vi "AES Decrypt.vi"(0 "Password.In":string, 2 "BitKeyType(256)":u16(ring)=256 items=["AES bit key 128"=128, "AES bit key 192"=192, "AES bit key 256"=256], 7 "EncryptedText.In":string, 11 "error in":errorcluster, 13 "nonce":u32=123456789) -> (8 "DecryptedText.Out":string, 15 "error out":errorcluster)   [LabVIEW 2011]
doc: "AES.Decrypt VI takes string encrypted with Advanced Encryption Standart (AES) and decrypts it into initial text. \nAES.Decrypt.vi allows reentrant execution.\n-------------------------------------------------------------------------------------------\nThis VI belongs to Server Lab tools at Labicom.net (www.labicom.net) project of remote and virtual laboratories, written by (c) Igor Titov, 2011."
panel:
  in  "Product information, copyright notice, list of conditions and disclaimer":string="Please visit http://www.labicom.net to learn about remote and virtual laboratories. With it's services and tools you can create remote and/or virtual laboratory and even make money on it.\n \nCopyright (C) 2011 Igor Titov igor.ev.titov@gmail.com\n\nAll rights reserved.\n\nRedistribution and use without modification, are permitted provided that the following conditions are met:\n\n    * Redistributions of source code must retain the above copyright notice, this list of conditions and the following disclaimer.\n    * Redistributions of source code and in binary form may be freely used in all sorts of projects (including commercial ones). It is not obligatory to place copyright notice, this list of conditions and the following disclaimer in your product but you must mention the source (www.labicom.net, Igor Titov) on the web-site of the product.\n    * Neither the name of \"Labicom\", \"labicom.net\", \"Igor Titov\", nor the names of its contributors may be used to endorse or promote products derived from this software without specific prior written permission (except in situations mentioned in the terms and conditions of use of the \"Labicom\").\n\nTHIS SOFTWARE IS PROVIDED BY THE COPYRIGHT HOLDERS AND CONTRIBUTORS \"AS IS\" AND ANY EXPRESS OR IMPLIED WARRANTIES, INCLUDING, BUT NOT LIMITED TO, THE IMPLIED WARRANTIES OF MERCHANTABILITY AND FITNESS FOR A PARTICULAR PURPOSE ARE DISCLAIMED. IN NO EVENT SHALL THE COPYRIGHT OWNER OR CONTRIBUTORS BE LIABLE FOR ANY DIRECT, INDIRECT, INCIDENTAL, SPECIAL, EXEMPLARY, OR CONSEQUENTIAL DAMAGES (INCLUDING, BUT NOT LIMITED TO, PROCUREMENT OF SUBSTITUTE GOODS OR SERVICES; LOSS OF USE, DATA, OR PROFITS; OR BUSINESS INTERRUPTION) HOWEVER CAUSED AND ON ANY THEORY OF LIABILITY, \nWHETHER IN CONTRACT, STRICT LIABILITY, OR TORT (INCLUDING NEGLIGENCE OR OTHERWISE) ARISING IN ANY WAY OUT OF THE USE OF THIS SOFTWARE, EVEN IF ADVISED OF THE POSSIBILITY OF SUCH DAMAGE. "
  in  "Decipher Phases":enum16{"Logical Shifts", "Combine Bytes"}(ring)
  in  "Decrypt Phases":enum16{"Init", "Decipher"}(ring)
  out "unsigned byte.utf8":u8[](array[numeric])
  out "unsigned byte.text":u8[](array[numeric])
  out "plaintxtByte":i32[](array[numeric])
  out "ciphertextArr":string[](array[string])
  out "ct":string[](array[string])
  out "nBlocks":i32
  out "cipherCntr":u16[](array[numeric])
  in  "0x100000000":u64=4294967296 format="%.0x"
  in  "blockSize":i32=16
  out "keySchedule":u32[](array[numeric])
  out "ctrTxt":string
  out "counterBlock":u32[](array[numeric])
  out "nonceSec":u32
  out "nonceMs":u32
  out "pwBytes":u32[](array[numeric])
  out "nBytes":i32
  # "Virtual & Remote Laboratories\nwww.labicom.net"
  # "Real lab at YOUR home"
  # "Number of bits used in the key (256 by default).\nThe longer a key, the higher level of protection\nat expence of processor and RAM usage."
  # "Advanced Encryption Standart (AES)\nAES.Decrypt 1.0"
  # "Receives Password in String format (plain text)"
  # "Receives encrypted text needed to be decrypted"
  # "Decrypted (plain) text"
  # "o?e?Ae§Oo??)y?B,UoV\"\nQoyµAv"
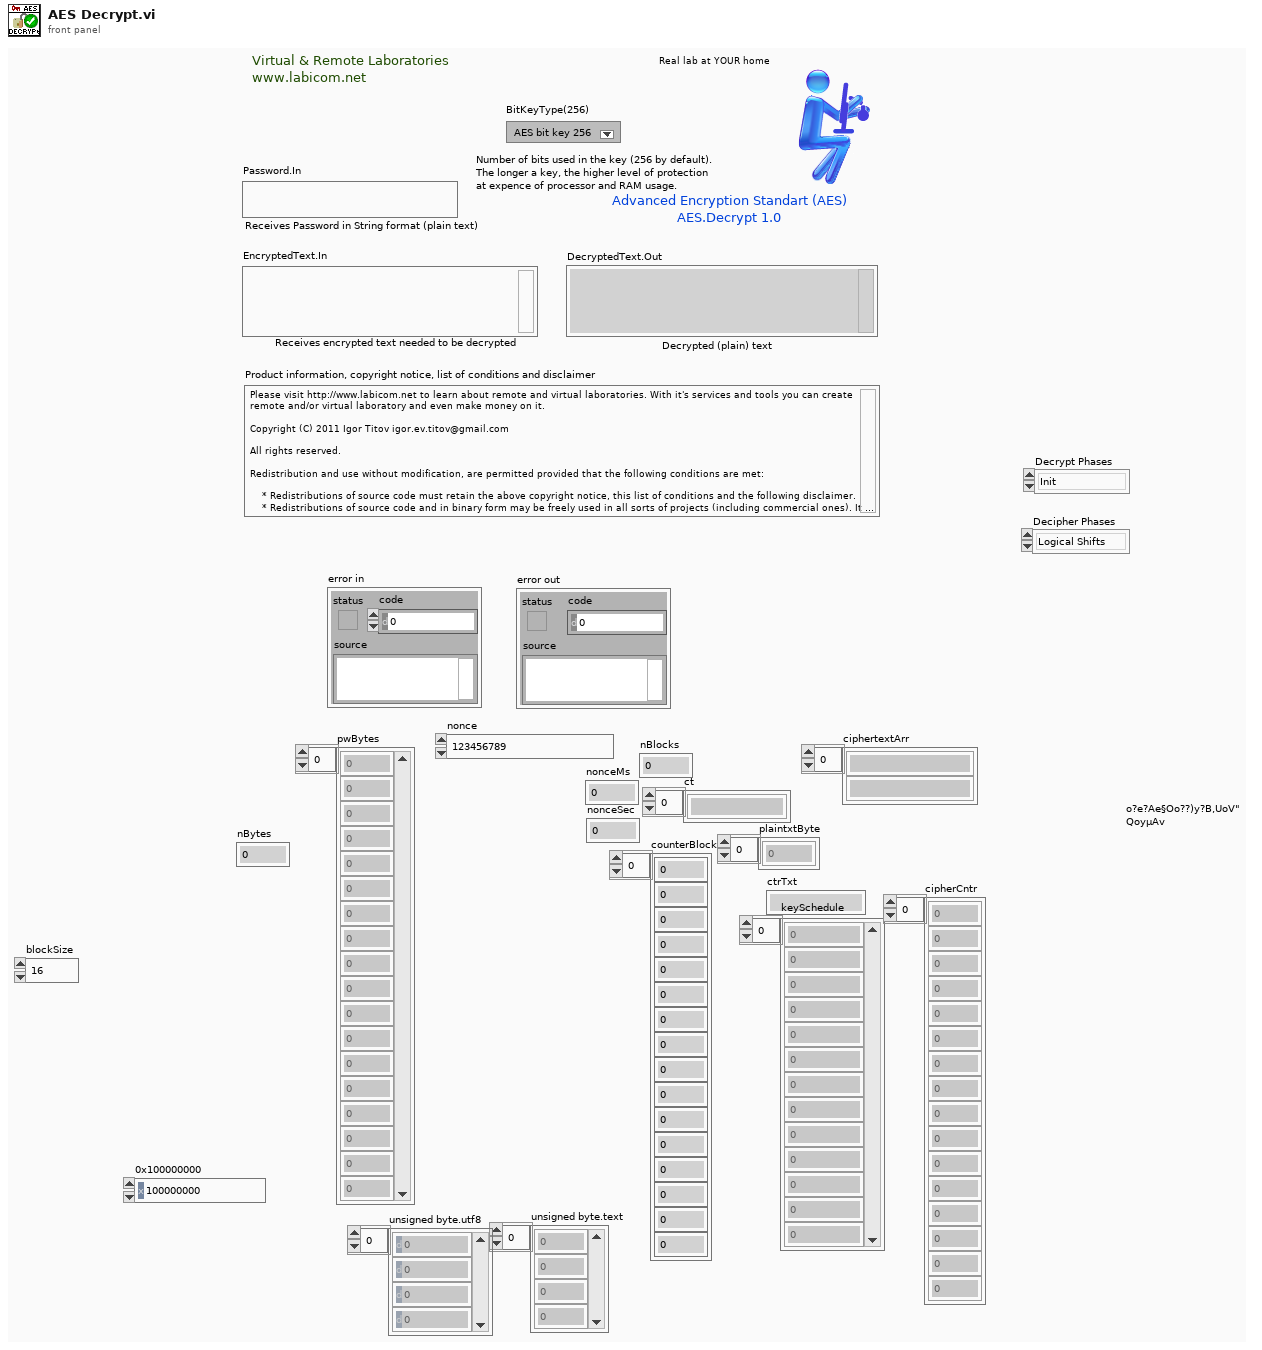
[diagram p1: front panel]
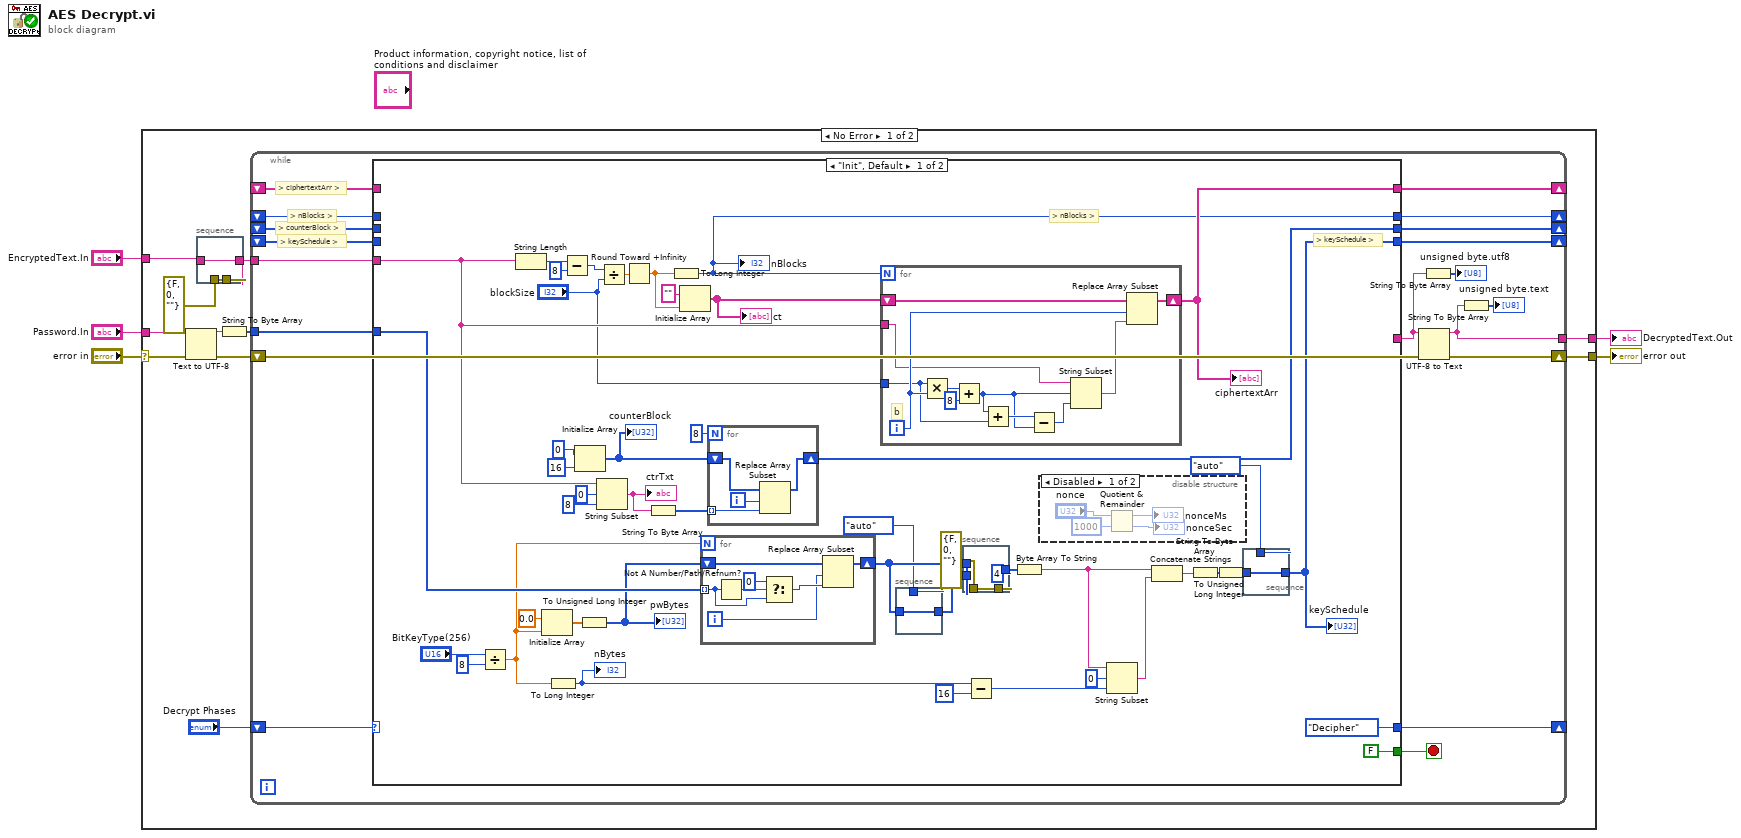
[diagram p0: block diagram]
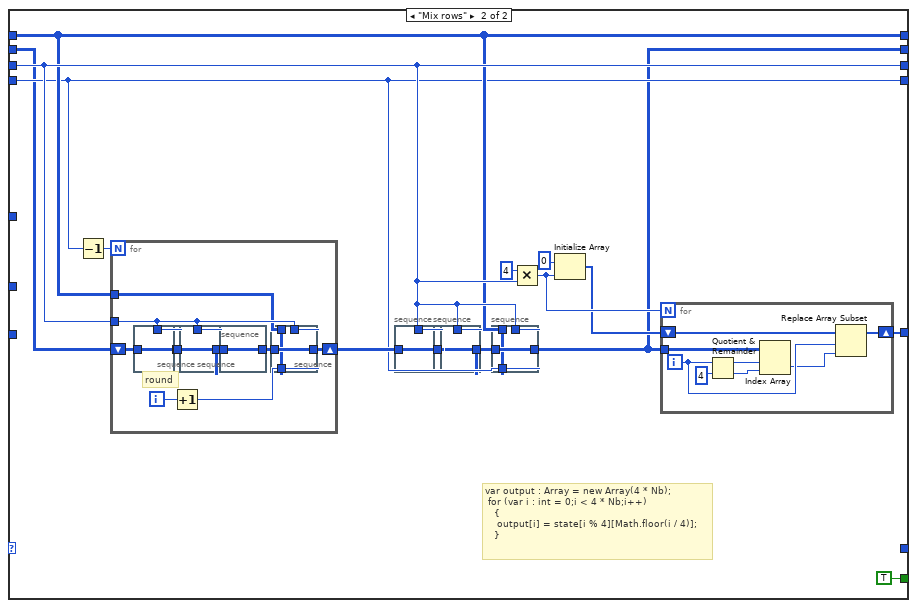
[diagram p2: hidden frame]
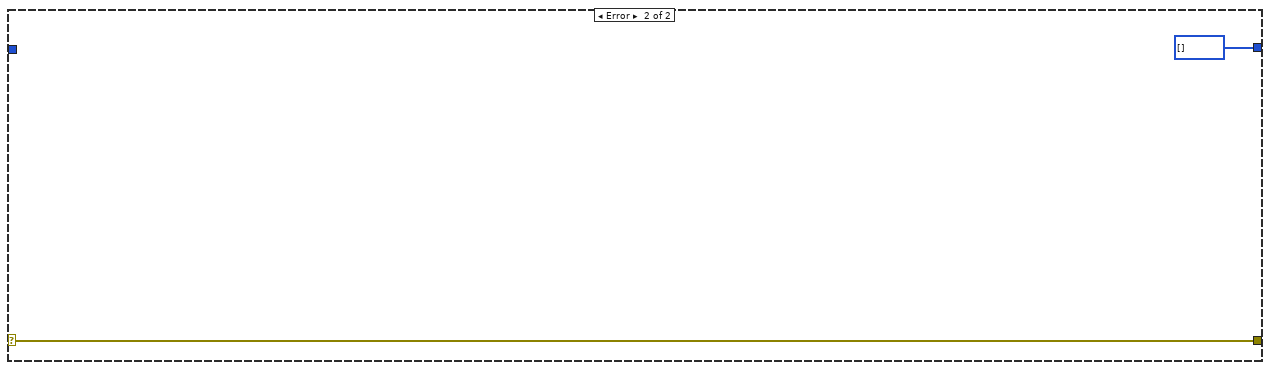
[diagram p3: hidden frame]
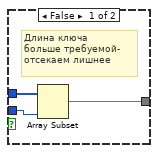
[diagram p4: hidden frame]
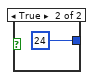
[diagram p5: hidden frame]
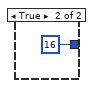
[diagram p6: hidden frame]
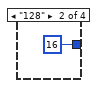
[diagram p7: hidden frame]
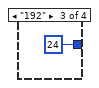
[diagram p8: hidden frame]
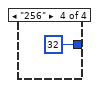
[diagram p9: hidden frame]
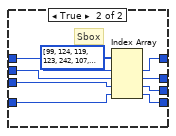
[diagram p10: hidden frame]
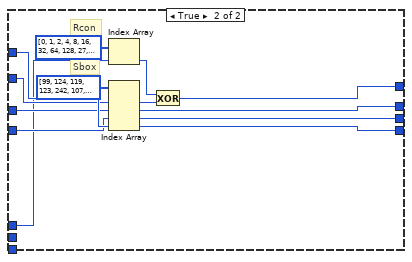
[diagram p11: hidden frame]
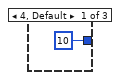
[diagram p12: hidden frame]
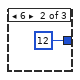
[diagram p13: hidden frame]
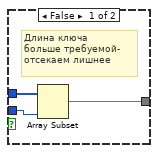
[diagram p14: hidden frame]
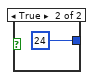
[diagram p15: hidden frame]
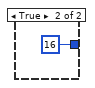
[diagram p16: hidden frame]
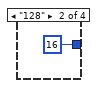
[diagram p17: hidden frame]
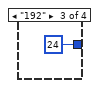
[diagram p18: hidden frame]
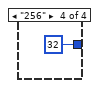
[diagram p19: hidden frame]
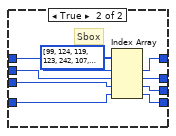
[diagram p20: hidden frame]
diagram:
  n1 = case shown="No Error" "error in" {
    selector: "error in" -> [w7 w1165]
    tunnel: [w12 w1165] -> w4
    tunnel: "EncryptedText.In" -> [w10 _]
    tunnel: "Password.In" -> [w9 _]
    tunnel: [w8 "" ("text")] -> w1
    frame No Error {
      n2 = Text to UTF-8(8:w7, 11:w9) -> (0:w11:errorcluster, 3:w15:string)
      n3 = stacked-sequence {
        tunnel: w10 -> [w28]
        tunnel: [w27] -> w13
        tunnel: errorcluster {"status"=FALSE, "code"=0, "source"=""} ("error in (no error)") -> [w35]
        tunnel: [w40] -> _
        frame #0 {
          w42 = TRUE ("replace all? (F)")
          w25 = 8 ("y")
          n4 = Search and Replace String(replace all?=w42, input string=w28, search string="\r" ("replace string (\"\")"), replace string="", error in=w35) -> (result string=w32:string, error out=w34:errorcluster)  [unwired: 5 out]
          n5 = Search and Replace String(replace all?=w42, input string=w32, search string="\n" ("replace string (\"\")"), replace string="", error in=w34) -> (result string=w38:string, error out=w39:errorcluster)  [unwired: 5 out]
          n6 = Search and Replace String(replace all?=w42, input string=w38, search string=" " ("replace string (\"\")"), replace string="", error in=w39) -> (result string=w41:string, error out=w40:errorcluster)  [unwired: 5 out]
          n7 = Match Pattern(string=w41, regular expression="=") -> (before substring=w20:string)  [unwired: 4 out]
          n8 = String Length(string=w20) -> (length=w17:i32)
          n9 = for {
            N: w17 -> [_]
            tunnel: w20 -> [w63]
            tunnel: "ABCDEFGHIJKLMNOPQRSTUVWXYZabcdefghijklmnopqrstuvwxyz0123456789+/" -> [w60]
            shift-right: [w53] -> w24
            shift-left: bool[] [] -> [w52]
            i -> [w61]
            n10 = String Subset(string=w63, offset (0)=w61, length (rest)=1 ("length (rest)")) -> (substring=w59:string)
            n11 = Match Pattern(string=w60, regular expression=w59) -> (offset past match=w58:i32)  [unwired: 1 in, 3 out]
            n12 = Decrement(x=w58) -> (x-1=w57:i32)
            n13 = Number To Boolean Array(number=w57) -> (Boolean array=w56:bool[])
            n14 = Array Subset(array=w56, length=6) -> (w54:bool[])  [unwired: 1 in]
            n15 = Reverse 1D Array(array=w54) -> (reversed array=w51:bool[])
            n16 = Build Array (concatenate)(w52, w51) -> (w53:bool[])
          }
          n17 = Array Size(array=w24) -> (size(s)=w22:i32)
          n18 = Quotient & Remainder(x=w22, y=w25) -> (floor(x/y)=w23:i32)  [unwired: 1 out]
          n19 = for {
            N: w23 -> [_]
            tunnel: w24 -> [w50]
            tunnel: w25 -> [w49]
            tunnel: [w45] -> w26 mode=indexing
            i -> [w48]
            n20 = Multiply(x=w48, y=w49) -> (x*y=w43:i32)
            n21 = Array Subset(array=w50, index=w43, length=w49) -> (w47:bool[])
            n22 = Reverse 1D Array(array=w47) -> (reversed array=w44:bool[])
            n23 = Boolean Array To Number(Boolean array=w44) -> (number=w46:u32)
            n24 = To Unsigned Byte Integer(number=w46) -> (unsigned 8bit integer=w45:u8)
          }
          n25 = Byte Array To String(unsigned byte array=w26) -> (string=w27:string)
        }
      }
      n26 = String To Byte Array(string=w15) -> (unsigned byte array=w14:u8[])
      n27 = while {
        shift-right: [w70] -> _
        shift-left: "Decrypt Phases" -> [w82]
        tunnel: w14 -> [w81]
        tunnel: w13 -> [w80]
        shift-right: [w78] -> _
        shift-left: _ -> [w77]
        shift-right: [w76] -> _
        shift-left: _ -> [w75]
        shift-right: [w74] -> _
        shift-left: _ -> [w73]
        shift-right: [w72] -> _
        shift-left: _ -> [w71]
        tunnel: [w66] -> w8
        shift-right: [w65] -> w12
        shift-left: w11 -> [w64]
        stop <- w79 stop-if-true
        # "> keySchedule >"
        # "> counterBlock >"
        # "> nBlocks >"
        # "> ciphertextArr >"
        n28 = case shown="\"Init\", Default" w82 {
          tunnel: w81 -> [w112 _]
          tunnel: w80 -> [w94 _]
          tunnel: [FALSE TRUE] -> w79
          tunnel: [w93 w758] -> w78
          tunnel: w77 -> [_ w758]
          tunnel: [w91 w759] -> w76
          tunnel: w75 -> [_ w759]
          tunnel: [w90 w760] -> w74
          tunnel: w73 -> [_ w760]
          tunnel: [w89 w762] -> w72
          tunnel: w71 -> [_ w762]
          tunnel: [enum16{"Init", "Decipher"}."Decipher" ("Decrypt Phases") _] -> w70
          tunnel: [_ w757] -> w67
          frame "Init", Default {
            # "> keySchedule >"
            # "> nBlocks >"
            n29 = Divide(x="BitKeyType(256)", y=u16 8) -> (x/y=w99:dbl)
            n30 = String Length(string=w94) -> (length=w121:i32)
            n31 = Initialize Array(0.0 ("element"), w99) -> (w111:dbl[])
            n32 = To Long Integer(number=w99) -> (32bit integer=w98:i32)
            "nBytes" <- w98
            n33 = Subtract(x=w121, y=8) -> (x-y=w119:i32)
            n34 = Initialize Array(u32 0 ("y"), 16 ("dimension size")) -> (w109:u32[])
            "counterBlock" <- w109
            n35 = To Unsigned Long Integer(number=w111) -> (unsigned 32bit integer=w110:u32[])
            "pwBytes" <- w110
            n36 = String Subset(string=w94, offset (0)=0, length (rest)=8 ("length (rest)")) -> (substring=w115:string)
            "ctrTxt" <- w115
            n37 = Divide(x=w119, y="blockSize") -> (x/y=w118:dbl)
            n38 = Round Toward +Infinity(x=w118) -> (ceil(x): smallest int >= x=w97:dbl)
            n39 = String To Byte Array(string=w115) -> (unsigned byte array=w116:u8[])
            n40 = To Long Integer(number=w97) -> (32bit integer=w91:i32)
            "nBlocks" <- w91
            n41 = Initialize Array("", w97) -> (w96:string[])
            "ct" <- w96
            n42 = for {
              N: w99 -> [_]
              tunnel: w112 -> [w751] mode=indexing
              shift-right: [w749] -> w100
              shift-left: w110 -> [w750]
              i -> [w753]
              n43 = Not A Number/Path/Refnum?(number/path/refnum=w751) -> (NaN/Path/Refnum?=w755:bool)
              n44 = Select(t=0 ("f"), s=w755, f=w751) -> (s? t:f=w754:i32)
              n45 = Replace Array Subset(array=w750, new element=w754, index=w753) -> (w749:u32[])
            }
            n46 = for {
              N: 8 -> [_]
              tunnel: w116 -> [w748] mode=indexing
              shift-right: [w745] -> w90
              shift-left: w109 -> [w746]
              i -> [w747]
              n47 = Replace Array Subset(array=w746, new element=w748, index=w747) -> (w745:u32[])
            }
            n48 = for {
              N: w91 -> [_]
              shift-right: [w736] -> w93
              shift-left: w96 -> [w737]
              tunnel: w94 -> [w735]
              tunnel: "blockSize" -> [w734]
              i -> [w742]
              # "b"
              n49 = Multiply(x=w734, y=w742) -> (x*y=w744:i32)
              n50 = Add(x=w744, y=8) -> (x+y=w739:i32)
              n51 = Add(x=w739, y=w734) -> (x+y=w740:i32)
              n52 = Subtract(x=w740, y=w739) -> (x-y=w738:i32)
              n53 = String Subset(string=w735, offset (0)=w739, length (rest)=w738) -> (substring=w741:string)
              n54 = Replace Array Subset(array=w737, new element=w741, index=w742) -> (w736:string[])
            }
            "ciphertextArr" <- w93
            n55 = stacked-sequence {
              tunnel: enum16{"128", "192", "256", "auto"}."auto" ("Mode (auto)") -> [w464]
              tunnel: w100 -> [w469]
              tunnel: [w470] -> w101
              frame #0 {
                n56 = Array Size(array=w469) -> (size(s)=w465:i32)
                n57 = case shown="\"auto\", Default" w464 {
                  tunnel: w465 -> [w479 _ _ _]
                  tunnel: [w480 16 24 32] -> w467
                  frame "auto", Default {
                    n58 = Less Or Equal?(x=w479, y=16) -> (x <= y?=w481:bool)
                    n59 = case shown="False" w481 {
                      tunnel: [w483 16] -> w480
                      tunnel: w479 -> [w486 _]
                      frame False {
                        n60 = Less Or Equal?(x=w486, y=24) -> (x <= y?=w484:bool)
                        n61 = case shown="False" w484 {
                          tunnel: [32 ("y") 24 ("y")] -> w483
                          frame False {
                          }
                          frame True {
                          }
                        }
                      }
                      frame True {
                      }
                    }
                  }
                  frame "128" {
                  }
                  frame "192" {
                  }
                  frame "256" {
                  }
                }
                n62 = Less?(x=w465, y=w467) -> (x < y?=w466:bool)
                n63 = case shown="True" w466 {
                  tunnel: w469 -> [w473 w474]
                  tunnel: w467 -> [w472 w478]
                  tunnel: [w471 w476] -> w468
                  frame False {
                    # "Длина ключа\nбольше требуемой-\nотсекаем лишнее"
                    n64 = Array Subset(array=w473, length=w472) -> (w471:u32[])  [unwired: 1 in]
                  }
                  frame True {
                    # "Длина ключа\nменьше требуемой-\nдополняем нулями"
                    n65 = Initialize Array(u32 0, w478) -> (w477:u32[])
                    n66 = Replace Array Subset(array=w477, new element=w474) -> (w476:u32[])  [unwired: 1 in]
                  }
                }
                n67 = Array Size(array=w468) -> (size(s)=w463:i32)
                n68 = Logical Shift(y=i8 -2, x=w463) -> (x << y=w456:i32)
                n69 = case shown="8" w456 {
                  tunnel: [10 12 14] -> w453
                  frame 4, Default {
                  }
                  frame 6 {
                  }
                  frame 8 {
                  }
                }
                n70 = Increment(x=w453) -> (x+1=w454:i32)
                n71 = Multiply(x=4, y=w454) -> (x*y=w460:i32)
                n72 = Logical Shift(y=i8 2, x=w460) -> (x << y=w459:i32)
                n73 = Initialize Array(u32 0 ("element"), w459) -> (w461:u32[])
                n74 = Replace Array Subset(array=w461, new element=w468) -> (w462:u32[])  [unwired: 1 in]
                n75 = while {
                  tunnel: w460 -> [w545]
                  tunnel: w456 -> [w525]
                  shift-right: [w502] -> w470
                  shift-left: w462 -> [w526]
                  tunnel: w467 -> [w524]
                  i -> [w546]
                  stop <- w544 continue-if-true
                  n76 = Add(x=w525, y=w546) -> (x+y=w528:i32)
                  n77 = Less?(x=w528, y=w545) -> (x < y?=w544:bool)
                  n78 = Quotient & Remainder(x=w528, y=w525) -> (x-y*floor(x/y)=w533:i32, floor(x/y)=w527:i32)
                  n79 = Logical Shift(y=i8 2, x=w528) -> (x << y=w497:i32)
                  n80 = Equal To 0?(x=w533) -> (x = 0?=w534:bool)
                  n81 = Subtract(x=w497, y=4) -> (x-y=w538:i32)
                  n82 = Subtract(x=w497, y=3) -> (x-y=w537:i32)
                  n83 = Subtract(x=w497, y=2) -> (x-y=w536:i32)
                  n84 = Subtract(x=w497, y=1) -> (x-y=w535:i32)
                  n85 = Index Array(array=w526, index #1=w538, index #2=w537, index #3=w536, index #4=w535) -> (element #1=w532:u32, element #2=w531:u32, element #3=w530:u32, element #4=w529:u32)
                  n86 = case shown="False" w534 {
                    tunnel: w525 -> [w561 _]
                    tunnel: w533 -> [w559 _]
                    tunnel: w532 -> [w554 w587]
                    tunnel: w531 -> [w553 w586]
                    tunnel: w530 -> [w552 w585]
                    tunnel: w529 -> [w551 w584]
                    tunnel: w527 -> [_ w583]
                    tunnel: [w550 w580] -> w506
                    tunnel: [w549 w579] -> w505
                    tunnel: [w548 w578] -> w504
                    tunnel: [w547 w577] -> w503
                    frame False {
                      n87 = Greater?(x=w561, y=6) -> (0:w557:bool)
                      n88 = Equal?(x=w559, y=4) -> (x = y?=w556:bool)
                      n89 = And(x=w557, y=w556) -> (x .and. y?=w555:bool)
                      n90 = case shown="False" w555 {
                        tunnel: w554 -> [w565 w574]
                        tunnel: w553 -> [w564 w573]
                        tunnel: w552 -> [w563 w572]
                        tunnel: w551 -> [w562 w571]
                        tunnel: [w565 w570] -> w550
                        tunnel: [w564 w569] -> w549
                        tunnel: [w563 w568] -> w548
                        tunnel: [w562 w567] -> w547
                        frame False {
                        }
                        frame True {
                          # "Sbox"
                          n91 = Index Array(array=u32[] [99, 124, 119, 123, 242, 107, 111, 197, 48, 1, 103, 43, 254, 215, 171, 118, 202, 130, 201, 125, 250, 89, 71, 240, 173, 212, 162, 175, 156, 164, 114, 192, 183, 253, 147, 38, 54, 63, 247, 204, 52, 165, 229, 241, 113, 216, 49, 21, 4, 199, 35, 195, 24, 150, 5, 154, 7, 18, 128, 226, 235, 39, 178, 117, 9, 131, 44, 26, 27, 110, 90, 160, 82, 59, 214, 179, 41, 227, 47, 132, 83, 209, 0, 237, 32, 252, 177, 91, 106, 203, 190, 57, 74, 76, 88, 207, 208, 239, 170, 251, 67, 77, 51, 133, 69, 249, 2, 127, 80, 60, 159, 168, 81, 163, 64, 143, 146, 157, 56, 245, 188, 182, 218, 33, 16, 255, 243, 210, 205, 12, 19, 236, 95, 151, 68, 23, 196, 167, 126, 61, 100, 93, 25, 115, 96, 129, 79, 220, 34, 42, 144, 136, 70, 238, 184, 20, 222, 94, 11, 219, 224, 50, 58, 10, 73, 6, 36, 92, 194, 211, 172, 98, 145, 149, 228, 121, 231, 200, 55, 109, 141, 213, 78, 169, 108, 86, 244, 234, 101, 122, 174, 8, 186, 120, 37, 46, 28, 166, 180, 198, 232, 221, 116, 31, 75, 189, 139, 138, 112, 62, 181, 102, 72, 3, 246, 14, 97, 53, 87, 185, 134, 193, 29, 158, 225, 248, 152, 17, 105, 217, 142, 148, 155, 30, 135, 233, 206, 85, 40, 223, 140, 161, 137, 13, 191, 230, 66, 104, 65, 153, 45, 15, 176, 84, 187, 22] ("Sbox"), index #1=w574, index #2=w573, index #3=w572, index #4=w571) -> (element #1=w570:u32, element #2=w569:u32, element #3=w568:u32, element #4=w567:u32)
                        }
                      }
                    }
                    frame True {
                      # "Sbox"
                      # "Rcon"
                      n92 = Index Array(array=u32[] [0, 1, 2, 4, 8, 16, 32, 64, 128, 27, 54] ("Rcon"), index=w583) -> (element=w582:u32)
                      n93 = Index Array(array=u32[] [99, 124, 119, 123, 242, 107, 111, 197, 48, 1, 103, 43, 254, 215, 171, 118, 202, 130, 201, 125, 250, 89, 71, 240, 173, 212, 162, 175, 156, 164, 114, 192, 183, 253, 147, 38, 54, 63, 247, 204, 52, 165, 229, 241, 113, 216, 49, 21, 4, 199, 35, 195, 24, 150, 5, 154, 7, 18, 128, 226, 235, 39, 178, 117, 9, 131, 44, 26, 27, 110, 90, 160, 82, 59, 214, 179, 41, 227, 47, 132, 83, 209, 0, 237, 32, 252, 177, 91, 106, 203, 190, 57, 74, 76, 88, 207, 208, 239, 170, 251, 67, 77, 51, 133, 69, 249, 2, 127, 80, 60, 159, 168, 81, 163, 64, 143, 146, 157, 56, 245, 188, 182, 218, 33, 16, 255, 243, 210, 205, 12, 19, 236, 95, 151, 68, 23, 196, 167, 126, 61, 100, 93, 25, 115, 96, 129, 79, 220, 34, 42, 144, 136, 70, 238, 184, 20, 222, 94, 11, 219, 224, 50, 58, 10, 73, 6, 36, 92, 194, 211, 172, 98, 145, 149, 228, 121, 231, 200, 55, 109, 141, 213, 78, 169, 108, 86, 244, 234, 101, 122, 174, 8, 186, 120, 37, 46, 28, 166, 180, 198, 232, 221, 116, 31, 75, 189, 139, 138, 112, 62, 181, 102, 72, 3, 246, 14, 97, 53, 87, 185, 134, 193, 29, 158, 225, 248, 152, 17, 105, 217, 142, 148, 155, 30, 135, 233, 206, 85, 40, 223, 140, 161, 137, 13, 191, 230, 66, 104, 65, 153, 45, 15, 176, 84, 187, 22] ("Sbox"), index #1=w586, index #2=w585, index #3=w584, index #4=w587) -> (element #1=w581:u32, element #2=w579:u32, element #3=w578:u32, element #4=w577:u32)
                      n94 = Exclusive Or(1:w581, 2:w582) -> (0:w580:u32)
                    }
                  }
                  n95 = Subtract(x=w497, y=w524) -> (x-y=w523:i32)
                  n96 = Add(x=w523, y=0) -> (x+y=w518:i32)
                  n97 = Add(x=w523, y=1) -> (x+y=w517:i32)
                  n98 = Add(x=w523, y=2) -> (x+y=w516:i32)
                  n99 = Add(x=w523, y=3) -> (x+y=w515:i32)
                  n100 = Index Array(array=w526, index #1=w518, index #2=w517, index #3=w516, index #4=w515) -> (element #1=w514:u32, element #2=w513:u32, element #3=w512:u32, element #4=w511:u32)
                  n101 = Exclusive Or(1:w506, 2:w514) -> (0:w510:u32)
                  n102 = Exclusive Or(1:w505, 2:w513) -> (0:w509:u32)
                  n103 = Exclusive Or(1:w504, 2:w512) -> (0:w508:u32)
                  n104 = Exclusive Or(1:w503, 2:w511) -> (0:w507:u32)
                  n105 = Add(x=w497, y=0) -> (x+y=w496:i32)
                  n106 = Add(x=w497, y=1) -> (x+y=w495:i32)
                  n107 = Add(x=w497, y=2) -> (x+y=w494:i32)
                  n108 = Add(x=w497, y=3) -> (x+y=w493:i32)
                  n109 = Replace Array Subset(array=w526, new element #1=w510, index #1=w496, new element #2=w509, index #2=w495, new element #3=w508, index #3=w494, new element #4=w507, index #4=w493) -> (w502:u32[])
                }
              }
            }
            n110 = stacked-sequence {
              tunnel: w100 -> [w131]
              tunnel: [w132] -> w102
              tunnel: w101 -> [w130]
              tunnel: errorcluster {"status"=FALSE, "code"=0, "source"=""} ("error in") -> [w128]
              tunnel: [w129] -> _
              frame #0 {
                n111 = case shown="No Error" w128 {
                  selector: w128 -> [_ w451]
                  tunnel: [_ w451] -> w129
                  tunnel: w130 -> [w137 _]
                  tunnel: w131 -> [w136 _]
                  tunnel: [w135 u16[] []] -> w132
                  tunnel: 4 ("Nb") -> [w134 _]
                  frame No Error {
                    n112 = while {
                      shift-right: [w141] -> _
                      shift-left: enum16{"Init", "Mix rows"}."Init" ("Cipher Phases") -> [w153]
                      tunnel: w137 -> [w152]
                      tunnel: w136 -> [w151]
                      shift-right: [w150] -> _
                      shift-left: _ -> [w149]
                      shift-right: [w148] -> _
                      shift-left: _ -> [w147]
                      shift-right: [w146] -> _
                      shift-left: _ -> [w145]
                      shift-right: [w144] -> _
                      shift-left: _ -> [w143]
                      tunnel: [w142] -> w135
                      tunnel: w134 -> [w139]
                      stop <- w140 stop-if-true
                      # "> Nr >"
                      # "> Nb >"
                      # "> State >"
                      # "> ExpandedKez(w)(2D) >"
                      n113 = case shown="\"Init\", Default" w153 {
                        tunnel: w152 -> [w166 _]
                        tunnel: w151 -> [w164 _]
                        tunnel: [w161 w214] -> w150
                        tunnel: w149 -> [_ w214]
                        tunnel: [w160 w207] -> w148
                        tunnel: w147 -> [_ w208]
                        tunnel: [w154 w215] -> w146
                        tunnel: w145 -> [_ w215]
                        tunnel: [w158 w213] -> w144
                        tunnel: w143 -> [_ w213]
                        tunnel: [_ w210] -> w142
                        tunnel: [enum16{"Init", "Mix rows"}."Mix rows" ("Cipher Phases") _] -> w141
                        tunnel: [FALSE TRUE] -> w140
                        tunnel: w139 -> [w154 _]
                        frame "Init", Default {
                          # "> Nb >"
                          # "> ExpandedKey(w)(2D) >"
                          # "> Nr >"
                          n114 = Reshape Array(w166, 60 ("dimension size"), 4 ("dimension size")) -> (w161:u32[][])
                          n115 = for {
                            N: 16 -> [_]
                            tunnel: w164 -> [w201]
                            shift-right: [w199] -> w162
                            shift-left: u16[][] [[0, 0, 0, 0], [0, 0, 0, 0], [0, 0, 0, 0], [0, 0, 0, 0]] ("State.Out") -> [w200]
                            i -> [w206]
                            n116 = Quotient & Remainder(x=w206, y=4) -> (x-y*floor(x/y)=w203:i32, floor(x/y)=w202:i32)
                            n117 = Index Array(array=w201, index=w206) -> (element=w204:u32)
                            n118 = Replace Array Subset(array=w200, new element=w204, index (row)=w203, index (col)=w202) -> (w199:u16[][])
                          }
                          n119 = Array Size(array=w161) -> (size(s)=w167:i32[])
                          n120 = Index Array(array=w167, index=0) -> (element=w170:i32)
                          n121 = Divide(x=w170, y=w154) -> (x/y=w169:dbl)
                          n122 = Decrement(x=w169) -> (x-1=w159:dbl)
                          n123 = To Long Integer(number=w159) -> (32bit integer=w158:i32)
                          n124 = stacked-sequence {
                            tunnel: w161 -> [w173]
                            tunnel: w154 -> [w175]
                            tunnel: w162 -> [w177]
                            tunnel: [w178] -> w160
                            tunnel: 0 ("rnd (0)") -> [w176]
                            frame #0 {
                              n125 = for {
                                N: 4 -> [_]
                                tunnel: w177 -> [w184]
                                tunnel: w173 -> [w183]
                                tunnel: w175 -> [w182]
                                tunnel: w176 -> [w181]
                                shift-right: [w179] -> w178
                                shift-left: w177 -> [w180]
                                i -> [w185]
                                # "w"
                                # "state"
                                # "r"
                                n126 = for {
                                N: w182 -> [_]
                                tunnel: w185 -> [w190]
                                tunnel: w184 -> [w193]
                                tunnel: w183 -> [w198]
                                tunnel: w181 -> [w197]
                                shift-right: [w186] -> w179
                                shift-left: w180 -> [w187]
                                i -> [w189]
                                # "c"
                                n127 = Multiply(x=w197, y=4) -> (x*y=w195:i32)
                                n128 = Add(x=w195, y=w189) -> (x+y=w194:i32)
                                n129 = Index Array(array=w193, index (row)=w190, index (col)=w189) -> (element=w192:u16)
                                n130 = Index Array(array=w198, index (row)=w194, index (col)=w190) -> (element=w191:u32)
                                n131 = Exclusive Or(1:w191, 2:w192) -> (0:w188:u32)
                                n132 = Replace Array Subset(array=w187, new element=w188, index (row)=w190, index (col)=w189) -> (w186:u16[][])
                                }
                              }
                            }
                          }
                        }
                        frame "Mix rows" {
                          # "var output : Array = new Array(4 * Nb); \n\tfor (var i : int = 0;i < 4 * Nb;i++)\n   {\n    output[i] = state[i % 4][Math.floor(i / 4)];\n\t\t\t}"
                          n133 = Decrement(x=w213) -> (x-1=w221:i32)
                          n134 = for {
                            N: w221 -> [_]
                            shift-right: [w304] -> w216
                            shift-left: w208 -> [w305]
                            tunnel: w215 -> [w303]
                            tunnel: w214 -> [w302]
                            i -> [w307]
                            # "round"
                            n135 = stacked-sequence {
                              tunnel: w303 -> [w311]
                              tunnel: w305 -> [w313]
                              tunnel: [w314] -> w310
                              frame #0 {
                                n136 = for {
                                N: 4 -> [_]
                                tunnel: w313 -> [w318]
                                shift-right: [w315] -> w314
                                shift-left: w313 -> [w317]
                                tunnel: w311 -> [w316]
                                i -> [w319]
                                # "> State.In >"
                                # "> State.Temp >"
                                # "r"
                                n137 = for {
                                N: w316 -> [_]
                                tunnel: w318 -> [w327]
                                tunnel: w319 -> [w324]
                                shift-right: [w320] -> w315
                                shift-left: w317 -> [w321]
                                i -> [w323]
                                # "Sbox"
                                # "s[r][c]"
                                # "c"
                                n138 = Index Array(array=w327, index (row)=w323, index (col)=w324) -> (element=w326:u16)
                                n139 = Index Array(array=u16[] [99, 124, 119, 123, 242, 107, 111, 197, 48, 1, 103, 43, 254, 215, 171, 118, 202, 130, 201, 125, 250, 89, 71, 240, 173, 212, 162, 175, 156, 164, 114, 192, 183, 253, 147, 38, 54, 63, 247, 204, 52, 165, 229, 241, 113, 216, 49, 21, 4, 199, 35, 195, 24, 150, 5, 154, 7, 18, 128, 226, 235, 39, 178, 117, 9, 131, 44, 26, 27, 110, 90, 160, 82, 59, 214, 179, 41, 227, 47, 132, 83, 209, 0, 237, 32, 252, 177, 91, 106, 203, 190, 57, 74, 76, 88, 207, 208, 239, 170, 251, 67, 77, 51, 133, 69, 249, 2, 127, 80, 60, 159, 168, 81, 163, 64, 143, 146, 157, 56, 245, 188, 182, 218, 33, 16, 255, 243, 210, 205, 12, 19, 236, 95, 151, 68, 23, 196, 167, 126, 61, 100, 93, 25, 115, 96, 129, 79, 220, 34, 42, 144, 136, 70, 238, 184, 20, 222, 94, 11, 219, 224, 50, 58, 10, 73, 6, 36, 92, 194, 211, 172, 98, 145, 149, 228, 121, 231, 200, 55, 109, 141, 213, 78, 169, 108, 86, 244, 234, 101, 122, 174, 8, 186, 120, 37, 46, 28, 166, 180, 198, 232, 221, 116, 31, 75, 189, 139, 138, 112, 62, 181, 102, 72, 3, 246, 14, 97, 53, 87, 185, 134, 193, 29, 158, 225, 248, 152, 17, 105, 217, 142, 148, 155, 30, 135, 233, 206, 85, 40, 223, 140, 161, 137, 13, 191, 230, 66, 104, 65, 153, 45, 15, 176, 84, 187, 22] ("Sbox"), index=w326) -> (element=w325:u16)
                                n140 = Replace Array Subset(array=w321, new element=w325, index (row)=w323, index (col)=w324) -> (w320:u16[][])
                                }
                                }
                              }
                            }
                            n141 = Increment(x=w307) -> (x+1=w306:i32)
                            n142 = stacked-sequence {
                              tunnel: w303 -> [w328]
                              tunnel: w310 -> [w330]
                              tunnel: [w331] -> w309
                              frame #0 {
                                n143 = for {
                                N: 3 -> [_]
                                tunnel: w330 -> [w341]
                                shift-right: [w337] -> w331
                                shift-left: w330 -> [w338]
                                tunnel: w328 -> [w332]
                                i -> [w340]
                                # "> t[c] >"
                                # "> State.In >"
                                # "> State.Temp >"
                                # "r"
                                n144 = Increment(x=w340) -> (x+1=w339:i32)
                                n145 = for {
                                N: 4 -> [_]
                                tunnel: w341 -> [w356]
                                tunnel: w339 -> [w352]
                                shift-right: [w348] -> w335
                                shift-left: i32[] [0, 0, 0, 0] ("t[c]") -> [w349]
                                tunnel: w332 -> [w354]
                                i -> [w351]
                                # "c"
                                n146 = Add(x=w352, y=w351) -> (x+y=w355:i32)
                                n147 = Quotient & Remainder(x=w355, y=w354) -> (x-y*floor(x/y)=w353:i32)  [unwired: 1 out]
                                n148 = Index Array(array=w356, index (row)=w352, index (col)=w353) -> (element=w350:u16)
                                n149 = Insert Into Array(array=w349, index=w351, new element=w350) -> (w348:i32[])
                                }
                                n150 = for {
                                N: 4 -> [_]
                                tunnel: w339 -> [w347]
                                shift-right: [w343] -> w337
                                shift-left: w338 -> [w344]
                                tunnel: w335 -> [w342]
                                i -> [w346]
                                # "c"
                                n151 = Index Array(array=w342, index=w346) -> (element=w345:i32)
                                n152 = Replace Array Subset(array=w344, new element=w345, index (row)=w347, index (col)=w346) -> (w343:u16[][])
                                }
                                }
                              }
                            }
                            n153 = stacked-sequence {
                              tunnel: w309 -> [w358]
                              tunnel: [w359] -> w308
                              frame #0 {
                                n154 = for {
                                N: 4 -> [_]
                                shift-right: [w403] -> w359
                                shift-left: w358 -> [w404]
                                tunnel: w358 -> [w405]
                                i -> [w406]
                                # "> b >"
                                # "> a >"
                                # "> State.In >"
                                # "> State.Temp >"
                                # "c"
                                n155 = To Unsigned Word Integer(number=i32[] [0, 0, 0, 0] ("t[c]")) -> (unsigned 16bit integer=w400:u16[])
                                n156 = To Unsigned Word Integer(number=i32[] [0, 0, 0, 0] ("t[c]")) -> (unsigned 16bit integer=w399:u16[])
                                n157 = for {
                                N: 4 -> [_]
                                tunnel: w405 -> [w423]
                                tunnel: w406 -> [w422]
                                shift-right: [w409] -> w398
                                shift-left: w400 -> [w410]
                                shift-right: [w407] -> w397
                                shift-left: w399 -> [w408]
                                i -> [w421]
                                # "s[i][c]"
                                # "i"
                                n158 = Index Array(array=w423, index (row)=w421, index (col)=w422) -> (element=w415:u16)
                                n159 = And(x=w415, y=u16 128 ("0x80")) -> (x .and. y?=w418:u16)
                                n160 = Logical Shift(y=i8 1, x=w415) -> (x << y=w412:u16)
                                n161 = Number To Boolean Array(number=w418) -> (Boolean array=w417:bool[])
                                n162 = Insert Into Array(array=w410, index=w421, new element=w415) -> (w409:u16[])
                                n163 = Exclusive Or(1:u16 283 ("0x011b"), 2:w412) -> (0:w413:u16)
                                n164 = Or Array Elements(Boolean array=w417) -> (logical OR=w416:bool)
                                n165 = Select(t=w413, s=w416, f=w412) -> (s? t:f=w420:u16)
                                n166 = Insert Into Array(array=w408, index=w421, new element=w420) -> (w407:u16[])
                                }
                                n167 = Index Array(array=w397, index #1=0 ("index"), index #2=1 ("index"), index #3=2 ("index"), index #4=3 ("index")) -> (element #1=w368:u16, element #2=w380:u16, element #3=w375:u16, element #4=w365:u16)
                                n168 = Index Array(array=w398, index #1=0 ("index"), index #2=1 ("index"), index #3=2 ("index"), index #4=3 ("index")) -> (element #1=w369:u16, element #2=w367:u16, element #3=w366:u16, element #4=w374:u16)
                                n169 = Exclusive Or(1:w367, 2:w368) -> (0:w387:u16)
                                n170 = Exclusive Or(1:w380, 2:w387) -> (0:w386:u16)
                                n171 = Exclusive Or(1:w367, 2:w369) -> (0:w378:u16)
                                n172 = Exclusive Or(1:w366, 2:w386) -> (0:w385:u16)
                                n173 = Exclusive Or(1:w368, 2:w369) -> (0:w372:u16)
                                n174 = Exclusive Or(1:w380, 2:w369) -> (0:w383:u16)
                                n175 = Exclusive Or(1:w375, 2:w378) -> (0:w377:u16)
                                n176 = Exclusive Or(1:w374, 2:w385) -> (0:w384:u16)
                                n177 = Exclusive Or(1:w367, 2:w372) -> (0:w371:u16)
                                n178 = Exclusive Or(1:w366, 2:w383) -> (0:w382:u16)
                                n179 = Exclusive Or(1:w374, 2:w377) -> (0:w376:u16)
                                n180 = Exclusive Or(1:w366, 2:w371) -> (0:w370:u16)
                                n181 = Exclusive Or(1:w375, 2:w382) -> (0:w381:u16)
                                n182 = Exclusive Or(1:w365, 2:w376) -> (0:w373:u16)
                                n183 = Exclusive Or(1:w365, 2:w370) -> (0:w364:u16)
                                n184 = Exclusive Or(1:w374, 2:w381) -> (0:w379:u16)
                                n185 = Replace Array Subset(array=w404, new element #1=w384, index (row) #1=0 ("disabled index (col)"), index (col) #1=w406, new element #2=w379, index (row) #2=1 ("disabled index (col)"), index (col) #2=w406, new element #3=w373, index (row) #3=2 ("disabled index (col)"), index (col) #3=w406, new element #4=w364, index (row) #4=3 ("disabled index (col)"), index (col) #4=w406) -> (w403:u16[][])
                                }
                              }
                            }
                            n186 = stacked-sequence {
                              tunnel: w302 -> [w424]
                              tunnel: w303 -> [w426]
                              tunnel: w308 -> [w428]
                              tunnel: [w429] -> w304
                              tunnel: w306 -> [w427]
                              frame #0 {
                                n187 = for {
                                N: 4 -> [_]
                                tunnel: w428 -> [w435]
                                tunnel: w424 -> [w434]
                                tunnel: w426 -> [w433]
                                tunnel: w427 -> [w432]
                                shift-right: [w430] -> w429
                                shift-left: w428 -> [w431]
                                i -> [w436]
                                # "w"
                                # "state"
                                # "r"
                                n188 = for {
                                N: w433 -> [_]
                                tunnel: w436 -> [w441]
                                tunnel: w435 -> [w444]
                                tunnel: w434 -> [w449]
                                tunnel: w432 -> [w448]
                                shift-right: [w437] -> w430
                                shift-left: w431 -> [w438]
                                i -> [w440]
                                # "c"
                                n189 = Multiply(x=w448, y=4) -> (x*y=w446:i32)
                                n190 = Add(x=w446, y=w440) -> (x+y=w445:i32)
                                n191 = Index Array(array=w444, index (row)=w441, index (col)=w440) -> (element=w443:u16)
                                n192 = Index Array(array=w449, index (row)=w445, index (col)=w441) -> (element=w442:u32)
                                n193 = Exclusive Or(1:w442, 2:w443) -> (0:w439:u32)
                                n194 = Replace Array Subset(array=w438, new element=w439, index (row)=w441, index (col)=w440) -> (w437:u16[][])
                                }
                                }
                              }
                            }
                          }
                          n195 = stacked-sequence {
                            tunnel: w215 -> [w277]
                            tunnel: w216 -> [w279]
                            tunnel: [w280] -> w220
                            frame #0 {
                              n196 = for {
                                N: 4 -> [_]
                                tunnel: w279 -> [w284]
                                shift-right: [w281] -> w280
                                shift-left: w279 -> [w283]
                                tunnel: w277 -> [w282]
                                i -> [w285]
                                # "> State.In >"
                                # "> State.Temp >"
                                # "r"
                                n197 = for {
                                N: w282 -> [_]
                                tunnel: w284 -> [w293]
                                tunnel: w285 -> [w290]
                                shift-right: [w286] -> w281
                                shift-left: w283 -> [w287]
                                i -> [w289]
                                # "Sbox"
                                # "s[r][c]"
                                # "c"
                                n198 = Index Array(array=w293, index (row)=w289, index (col)=w290) -> (element=w292:u16)
                                n199 = Index Array(array=u16[] [99, 124, 119, 123, 242, 107, 111, 197, 48, 1, 103, 43, 254, 215, 171, 118, 202, 130, 201, 125, 250, 89, 71, 240, 173, 212, 162, 175, 156, 164, 114, 192, 183, 253, 147, 38, 54, 63, 247, 204, 52, 165, 229, 241, 113, 216, 49, 21, 4, 199, 35, 195, 24, 150, 5, 154, 7, 18, 128, 226, 235, 39, 178, 117, 9, 131, 44, 26, 27, 110, 90, 160, 82, 59, 214, 179, 41, 227, 47, 132, 83, 209, 0, 237, 32, 252, 177, 91, 106, 203, 190, 57, 74, 76, 88, 207, 208, 239, 170, 251, 67, 77, 51, 133, 69, 249, 2, 127, 80, 60, 159, 168, 81, 163, 64, 143, 146, 157, 56, 245, 188, 182, 218, 33, 16, 255, 243, 210, 205, 12, 19, 236, 95, 151, 68, 23, 196, 167, 126, 61, 100, 93, 25, 115, 96, 129, 79, 220, 34, 42, 144, 136, 70, 238, 184, 20, 222, 94, 11, 219, 224, 50, 58, 10, 73, 6, 36, 92, 194, 211, 172, 98, 145, 149, 228, 121, 231, 200, 55, 109, 141, 213, 78, 169, 108, 86, 244, 234, 101, 122, 174, 8, 186, 120, 37, 46, 28, 166, 180, 198, 232, 221, 116, 31, 75, 189, 139, 138, 112, 62, 181, 102, 72, 3, 246, 14, 97, 53, 87, 185, 134, 193, 29, 158, 225, 248, 152, 17, 105, 217, 142, 148, 155, 30, 135, 233, 206, 85, 40, 223, 140, 161, 137, 13, 191, 230, 66, 104, 65, 153, 45, 15, 176, 84, 187, 22] ("Sbox"), index=w292) -> (element=w291:u16)
                                n200 = Replace Array Subset(array=w287, new element=w291, index (row)=w289, index (col)=w290) -> (w286:u16[][])
                                }
                              }
                            }
                          }
                          n201 = stacked-sequence {
                            tunnel: w215 -> [w248]
                            tunnel: w220 -> [w250]
                            tunnel: [w251] -> w219
                            frame #0 {
                              n202 = for {
                                N: 3 -> [_]
                                tunnel: w250 -> [w261]
                                shift-right: [w257] -> w251
                                shift-left: w250 -> [w258]
                                tunnel: w248 -> [w252]
                                i -> [w260]
                                # "> t[c] >"
                                # "> State.In >"
                                # "> State.Temp >"
                                # "r"
                                n203 = Increment(x=w260) -> (x+1=w259:i32)
                                n204 = for {
                                N: 4 -> [_]
                                tunnel: w261 -> [w276]
                                tunnel: w259 -> [w272]
                                shift-right: [w268] -> w255
                                shift-left: i32[] [0, 0, 0, 0] ("t[c]") -> [w269]
                                tunnel: w252 -> [w274]
                                i -> [w271]
                                # "c"
                                n205 = Add(x=w272, y=w271) -> (x+y=w275:i32)
                                n206 = Quotient & Remainder(x=w275, y=w274) -> (x-y*floor(x/y)=w273:i32)  [unwired: 1 out]
                                n207 = Index Array(array=w276, index (row)=w272, index (col)=w273) -> (element=w270:u16)
                                n208 = Insert Into Array(array=w269, index=w271, new element=w270) -> (w268:i32[])
                                }
                                n209 = for {
                                N: 4 -> [_]
                                tunnel: w259 -> [w267]
                                shift-right: [w263] -> w257
                                shift-left: w258 -> [w264]
                                tunnel: w255 -> [w262]
                                i -> [w266]
                                # "c"
                                n210 = Index Array(array=w262, index=w266) -> (element=w265:i32)
                                n211 = Replace Array Subset(array=w264, new element=w265, index (row)=w267, index (col)=w266) -> (w263:u16[][])
                                }
                              }
                            }
                          }
                          n212 = stacked-sequence {
                            tunnel: w214 -> [w222]
                            tunnel: w215 -> [w224]
                            tunnel: w219 -> [w226]
                            tunnel: [w227] -> w207
                            tunnel: w213 -> [w225]
                            frame #0 {
                              n213 = for {
                                N: 4 -> [_]
                                tunnel: w226 -> [w233]
                                tunnel: w222 -> [w232]
                                tunnel: w224 -> [w231]
                                tunnel: w225 -> [w230]
                                shift-right: [w228] -> w227
                                shift-left: w226 -> [w229]
                                i -> [w234]
                                # "w"
                                # "state"
                                # "r"
                                n214 = for {
                                N: w231 -> [_]
                                tunnel: w234 -> [w239]
                                tunnel: w233 -> [w242]
                                tunnel: w232 -> [w247]
                                tunnel: w230 -> [w246]
                                shift-right: [w235] -> w228
                                shift-left: w229 -> [w236]
                                i -> [w238]
                                # "c"
                                n215 = Multiply(x=w246, y=4) -> (x*y=w244:i32)
                                n216 = Add(x=w244, y=w238) -> (x+y=w243:i32)
                                n217 = Index Array(array=w242, index (row)=w239, index (col)=w238) -> (element=w241:u16)
                                n218 = Index Array(array=w247, index (row)=w243, index (col)=w239) -> (element=w240:u32)
                                n219 = Exclusive Or(1:w240, 2:w241) -> (0:w237:u32)
                                n220 = Replace Array Subset(array=w236, new element=w237, index (row)=w239, index (col)=w238) -> (w235:u16[][])
                                }
                              }
                            }
                          }
                          n221 = Multiply(x=4, y=w215) -> (x*y=w212:i32)
                          n222 = Initialize Array(u16 0 ("x"), w212) -> (w211:u16[])
                          n223 = for {
                            N: w212 -> [_]
                            shift-right: [w294] -> w210
                            shift-left: w211 -> [w295]
                            tunnel: w207 -> [w296]
                            i -> [w298]
                            n224 = Quotient & Remainder(x=w298, y=4) -> (x-y*floor(x/y)=w300:i32, floor(x/y)=w299:i32)
                            n225 = Index Array(array=w296, index (row)=w300, index (col)=w299) -> (element=w297:u16)
                            n226 = Replace Array Subset(array=w295, new element=w297, index=w298) -> (w294:u16[])
                          }
                        }
                      }
                    }
                  }
                  frame Error {
                  }
                }
              }
            }
            n227 = Subtract(x=w98, y=u8 16) -> (x-y=w106:i32)
            n228 = Byte Array To String(unsigned byte array=w102) -> (string=w103:string)
            n229 = disable-structure shown="Disabled" {
              frame Disabled {
                n230 = Quotient & Remainder(x="nonce", y=u32 1000) -> (x-y*floor(x/y)=→"nonceMs":u32, floor(x/y)=→"nonceSec":u32)
              }
              frame Enabled {
              }
            }
            n231 = String Subset(string=w103, offset (0)=0, length (rest)=w106) -> (substring=w107:string)
            n232 = Concatenate Strings(w103, w107) -> (w108:string)
            n233 = String To Byte Array(string=w108) -> (unsigned byte array=w87:u8[])
            n234 = To Unsigned Long Integer(number=w87) -> (unsigned 32bit integer=w86:u32[])
            n235 = stacked-sequence {
              tunnel: enum16{"128", "192", "256", "auto"}."auto" ("Mode (auto)") -> [w603]
              tunnel: w86 -> [w608]
              tunnel: [w609] -> w89
              frame #0 {
                n236 = Array Size(array=w608) -> (size(s)=w604:i32)
                n237 = case shown="\"auto\", Default" w603 {
                  tunnel: w604 -> [w618 _ _ _]
                  tunnel: [w619 16 24 32] -> w606
                  frame "auto", Default {
                    n238 = Less Or Equal?(x=w618, y=16) -> (x <= y?=w620:bool)
                    n239 = case shown="False" w620 {
                      tunnel: [w622 16] -> w619
                      tunnel: w618 -> [w625 _]
                      frame False {
                        n240 = Less Or Equal?(x=w625, y=24) -> (x <= y?=w623:bool)
                        n241 = case shown="False" w623 {
                          tunnel: [32 ("y") 24 ("y")] -> w622
                          frame False {
                          }
                          frame True {
                          }
                        }
                      }
                      frame True {
                      }
                    }
                  }
                  frame "128" {
                  }
                  frame "192" {
                  }
                  frame "256" {
                  }
                }
                n242 = Less?(x=w604, y=w606) -> (x < y?=w605:bool)
                n243 = case shown="True" w605 {
                  tunnel: w608 -> [w612 w613]
                  tunnel: w606 -> [w611 w617]
                  tunnel: [w610 w615] -> w607
                  frame False {
                    # "Длина ключа\nбольше требуемой-\nотсекаем лишнее"
                    n244 = Array Subset(array=w612, length=w611) -> (w610:u32[])  [unwired: 1 in]
                  }
                  frame True {
                    # "Длина ключа\nменьше требуемой-\nдополняем нулями"
                    n245 = Initialize Array(u32 0, w617) -> (w616:u32[])
                    n246 = Replace Array Subset(array=w616, new element=w613) -> (w615:u32[])  [unwired: 1 in]
                  }
                }
                n247 = Array Size(array=w607) -> (size(s)=w602:i32)
                n248 = Logical Shift(y=i8 -2, x=w602) -> (x << y=w595:i32)
                n249 = case shown="8" w595 {
                  tunnel: [10 12 14] -> w592
                  frame 4, Default {
                  }
                  frame 6 {
                  }
                  frame 8 {
                  }
                }
                n250 = Increment(x=w592) -> (x+1=w593:i32)
                n251 = Multiply(x=4, y=w593) -> (x*y=w599:i32)
                n252 = Logical Shift(y=i8 2, x=w599) -> (x << y=w598:i32)
                n253 = Initialize Array(u32 0 ("element"), w598) -> (w600:u32[])
                n254 = Replace Array Subset(array=w600, new element=w607) -> (w601:u32[])  [unwired: 1 in]
                n255 = while {
                  tunnel: w599 -> [w684]
                  tunnel: w595 -> [w664]
                  shift-right: [w641] -> w609
                  shift-left: w601 -> [w665]
                  tunnel: w606 -> [w663]
                  i -> [w685]
                  stop <- w683 continue-if-true
                  n256 = Add(x=w664, y=w685) -> (x+y=w667:i32)
                  n257 = Less?(x=w667, y=w684) -> (x < y?=w683:bool)
                  n258 = Quotient & Remainder(x=w667, y=w664) -> (x-y*floor(x/y)=w672:i32, floor(x/y)=w666:i32)
                  n259 = Logical Shift(y=i8 2, x=w667) -> (x << y=w636:i32)
                  n260 = Equal To 0?(x=w672) -> (x = 0?=w673:bool)
                  n261 = Subtract(x=w636, y=4) -> (x-y=w677:i32)
                  n262 = Subtract(x=w636, y=3) -> (x-y=w676:i32)
                  n263 = Subtract(x=w636, y=2) -> (x-y=w675:i32)
                  n264 = Subtract(x=w636, y=1) -> (x-y=w674:i32)
                  n265 = Index Array(array=w665, index #1=w677, index #2=w676, index #3=w675, index #4=w674) -> (element #1=w671:u32, element #2=w670:u32, element #3=w669:u32, element #4=w668:u32)
                  n266 = case shown="False" w673 {
                    tunnel: w664 -> [w700 _]
                    tunnel: w672 -> [w698 _]
                    tunnel: w671 -> [w693 w726]
                    tunnel: w670 -> [w692 w725]
                    tunnel: w669 -> [w691 w724]
                    tunnel: w668 -> [w690 w723]
                    tunnel: w666 -> [_ w722]
                    tunnel: [w689 w719] -> w645
                    tunnel: [w688 w718] -> w644
                    tunnel: [w687 w717] -> w643
                    tunnel: [w686 w716] -> w642
                    frame False {
                      n267 = Greater?(x=w700, y=6) -> (0:w696:bool)
                      n268 = Equal?(x=w698, y=4) -> (x = y?=w695:bool)
                      n269 = And(x=w696, y=w695) -> (x .and. y?=w694:bool)
                      n270 = case shown="False" w694 {
                        tunnel: w693 -> [w704 w713]
                        tunnel: w692 -> [w703 w712]
                        tunnel: w691 -> [w702 w711]
                        tunnel: w690 -> [w701 w710]
                        tunnel: [w704 w709] -> w689
                        tunnel: [w703 w708] -> w688
                        tunnel: [w702 w707] -> w687
                        tunnel: [w701 w706] -> w686
                        frame False {
                        }
                        frame True {
                          # "Sbox"
                          n271 = Index Array(array=u32[] [99, 124, 119, 123, 242, 107, 111, 197, 48, 1, 103, 43, 254, 215, 171, 118, 202, 130, 201, 125, 250, 89, 71, 240, 173, 212, 162, 175, 156, 164, 114, 192, 183, 253, 147, 38, 54, 63, 247, 204, 52, 165, 229, 241, 113, 216, 49, 21, 4, 199, 35, 195, 24, 150, 5, 154, 7, 18, 128, 226, 235, 39, 178, 117, 9, 131, 44, 26, 27, 110, 90, 160, 82, 59, 214, 179, 41, 227, 47, 132, 83, 209, 0, 237, 32, 252, 177, 91, 106, 203, 190, 57, 74, 76, 88, 207, 208, 239, 170, 251, 67, 77, 51, 133, 69, 249, 2, 127, 80, 60, 159, 168, 81, 163, 64, 143, 146, 157, 56, 245, 188, 182, 218, 33, 16, 255, 243, 210, 205, 12, 19, 236, 95, 151, 68, 23, 196, 167, 126, 61, 100, 93, 25, 115, 96, 129, 79, 220, 34, 42, 144, 136, 70, 238, 184, 20, 222, 94, 11, 219, 224, 50, 58, 10, 73, 6, 36, 92, 194, 211, 172, 98, 145, 149, 228, 121, 231, 200, 55, 109, 141, 213, 78, 169, 108, 86, 244, 234, 101, 122, 174, 8, 186, 120, 37, 46, 28, 166, 180, 198, 232, 221, 116, 31, 75, 189, 139, 138, 112, 62, 181, 102, 72, 3, 246, 14, 97, 53, 87, 185, 134, 193, 29, 158, 225, 248, 152, 17, 105, 217, 142, 148, 155, 30, 135, 233, 206, 85, 40, 223, 140, 161, 137, 13, 191, 230, 66, 104, 65, 153, 45, 15, 176, 84, 187, 22] ("Sbox"), index #1=w713, index #2=w712, index #3=w711, index #4=w710) -> (element #1=w709:u32, element #2=w708:u32, element #3=w707:u32, element #4=w706:u32)
                        }
                      }
                    }
                    frame True {
                      # "Sbox"
                      # "Rcon"
                      n272 = Index Array(array=u32[] [0, 1, 2, 4, 8, 16, 32, 64, 128, 27, 54] ("Rcon"), index=w722) -> (element=w721:u32)
                      n273 = Index Array(array=u32[] [99, 124, 119, 123, 242, 107, 111, 197, 48, 1, 103, 43, 254, 215, 171, 118, 202, 130, 201, 125, 250, 89, 71, 240, 173, 212, 162, 175, 156, 164, 114, 192, 183, 253, 147, 38, 54, 63, 247, 204, 52, 165, 229, 241, 113, 216, 49, 21, 4, 199, 35, 195, 24, 150, 5, 154, 7, 18, 128, 226, 235, 39, 178, 117, 9, 131, 44, 26, 27, 110, 90, 160, 82, 59, 214, 179, 41, 227, 47, 132, 83, 209, 0, 237, 32, 252, 177, 91, 106, 203, 190, 57, 74, 76, 88, 207, 208, 239, 170, 251, 67, 77, 51, 133, 69, 249, 2, 127, 80, 60, 159, 168, 81, 163, 64, 143, 146, 157, 56, 245, 188, 182, 218, 33, 16, 255, 243, 210, 205, 12, 19, 236, 95, 151, 68, 23, 196, 167, 126, 61, 100, 93, 25, 115, 96, 129, 79, 220, 34, 42, 144, 136, 70, 238, 184, 20, 222, 94, 11, 219, 224, 50, 58, 10, 73, 6, 36, 92, 194, 211, 172, 98, 145, 149, 228, 121, 231, 200, 55, 109, 141, 213, 78, 169, 108, 86, 244, 234, 101, 122, 174, 8, 186, 120, 37, 46, 28, 166, 180, 198, 232, 221, 116, 31, 75, 189, 139, 138, 112, 62, 181, 102, 72, 3, 246, 14, 97, 53, 87, 185, 134, 193, 29, 158, 225, 248, 152, 17, 105, 217, 142, 148, 155, 30, 135, 233, 206, 85, 40, 223, 140, 161, 137, 13, 191, 230, 66, 104, 65, 153, 45, 15, 176, 84, 187, 22] ("Sbox"), index #1=w725, index #2=w724, index #3=w723, index #4=w726) -> (element #1=w720:u32, element #2=w718:u32, element #3=w717:u32, element #4=w716:u32)
                      n274 = Exclusive Or(1:w720, 2:w721) -> (0:w719:u32)
                    }
                  }
                  n275 = Subtract(x=w636, y=w663) -> (x-y=w662:i32)
                  n276 = Add(x=w662, y=0) -> (x+y=w657:i32)
                  n277 = Add(x=w662, y=1) -> (x+y=w656:i32)
                  n278 = Add(x=w662, y=2) -> (x+y=w655:i32)
                  n279 = Add(x=w662, y=3) -> (x+y=w654:i32)
                  n280 = Index Array(array=w665, index #1=w657, index #2=w656, index #3=w655, index #4=w654) -> (element #1=w653:u32, element #2=w652:u32, element #3=w651:u32, element #4=w650:u32)
                  n281 = Exclusive Or(1:w645, 2:w653) -> (0:w649:u32)
                  n282 = Exclusive Or(1:w644, 2:w652) -> (0:w648:u32)
                  n283 = Exclusive Or(1:w643, 2:w651) -> (0:w647:u32)
                  n284 = Exclusive Or(1:w642, 2:w650) -> (0:w646:u32)
                  n285 = Add(x=w636, y=0) -> (x+y=w635:i32)
                  n286 = Add(x=w636, y=1) -> (x+y=w634:i32)
                  n287 = Add(x=w636, y=2) -> (x+y=w633:i32)
                  n288 = Add(x=w636, y=3) -> (x+y=w632:i32)
                  n289 = Replace Array Subset(array=w665, new element #1=w649, index #1=w635, new element #2=w648, index #2=w634, new element #3=w647, index #3=w633, new element #4=w646, index #4=w632) -> (w641:u32[])
                }
              }
            }
            "keySchedule" <- w89
          }
          frame "Decipher" {
            n290 = for {
              N: w759 -> [_]
              shift-right: [w770] -> _
              shift-left: w760 -> [w771]
              tunnel: w762 -> [w769]
              shift-right: [w768] -> _
              shift-left: _ -> [w767]
              tunnel: w758 -> [w766]
              shift-right: [w765] -> w757
              shift-left: "" -> [w764]
              i -> [w772]
              # "> keySchedule >"
              # "> ciphertextArr >"
              # "> plaintxt >"
              # "> cipherCntr >"
              # "> counterBlock >"
              # "b"
              n291 = while {
                tunnel: w772 -> [w784]
                shift-right: [w773] -> _
                shift-left: "Decipher Phases" -> [w775]
                shift-right: [w782] -> w770
                shift-left: w771 -> [w783]
                tunnel: w769 -> [w781]
                shift-right: [w780] -> w768
                shift-left: w767 -> [w778]
                tunnel: w766 -> [w779]
                shift-right: [w777] -> w765
                shift-left: w764 -> [w776]
                stop <- w774 stop-if-true
                n292 = case shown="\"Logical Shifts\", Default" w775 {
                  tunnel: w784 -> [w793 w1149]
                  tunnel: w783 -> [w792 w1145]
                  tunnel: [w791 w1145] -> w782
                  tunnel: w781 -> [w790 _]
                  tunnel: [w789 w1146] -> w780
                  tunnel: w779 -> [_ w1148]
                  tunnel: w778 -> [_ w1146]
                  tunnel: [w788 w1144] -> w777
                  tunnel: w776 -> [w788 w1143]
                  tunnel: [FALSE TRUE] -> w774
                  tunnel: [enum16{"Logical Shifts", "Combine Bytes"}."Combine Bytes" ("Decipher Phases") _] -> w773
                  frame "Logical Shifts", Default {
                    n293 = Increment(x=w793) -> (x+1=w795:i32)
                    n294 = for {
                      N: 4 -> [_]
                      tunnel: w793 -> [w1139]
                      tunnel: w795 -> [w1133]
                      shift-right: [w1120] -> w791
                      shift-left: w792 -> [w1121]
                      i -> [w1128]
                      # "c"
                      n295 = Multiply(x=w1128, y=-8 ("x")) -> (x*y=w1127:i32)
                      n296 = Divide(x=w1133, y="0x100000000") -> (x/y=w1130:dbl)
                      n297 = Multiply(x=-8, y=w1128) -> (x*y=w1132:i32)
                      n298 = Decrement(x=w1130) -> (x-1=w1126:dbl)
                      n299 = Logical Shift(y=w1132, x=w1139) -> (x << y=w1141:i32)
                      n300 = Logical Shift(y=w1127, x=w1126) -> (x << y=w1125:u32)
                      n301 = And(x=w1141, y=u16 255 ("0xff")) -> (x .and. y?=w1137:i32)
                      n302 = Subtract(x=15, y=w1128) -> (x-y=w1136:i32)
                      n303 = And(x=u16 255 ("0xff"), y=w1125) -> (x .and. y?=w1124:u32)
                      n304 = Subtract(x=w1136, y=4) -> (x-y=w1134:i32)
                      n305 = Replace Array Subset(array=w1121, new element #1=w1137, index #1=w1136, new element #2=w1124, index #2=w1134) -> (w1120:u32[])
                    }
                    n306 = stacked-sequence {
                      tunnel: w791 -> [w799]
                      tunnel: [w800] -> w789
                      tunnel: w790 -> [w798]
                      tunnel: errorcluster {"status"=FALSE, "code"=0, "source"=""} ("error in") -> [w796]
                      tunnel: [w797] -> _
                      frame #0 {
                        n307 = case shown="No Error" w796 {
                          selector: w796 -> [_ w1119]
                          tunnel: [_ w1119] -> w797
                          tunnel: w798 -> [w805 _]
                          tunnel: w799 -> [w804 _]
                          tunnel: [w803 u16[] []] -> w800
                          tunnel: 4 ("Nb") -> [w802 _]
                          frame No Error {
                            n308 = while {
                              shift-right: [w809] -> _
                              shift-left: enum16{"Init", "Mix rows"}."Init" ("Cipher Phases") -> [w821]
                              tunnel: w805 -> [w820]
                              tunnel: w804 -> [w819]
                              shift-right: [w818] -> _
                              shift-left: _ -> [w817]
                              shift-right: [w816] -> _
                              shift-left: _ -> [w815]
                              shift-right: [w814] -> _
                              shift-left: _ -> [w813]
                              shift-right: [w812] -> _
                              shift-left: _ -> [w811]
                              tunnel: [w810] -> w803
                              tunnel: w802 -> [w807]
                              stop <- w808 stop-if-true
                              # "> Nr >"
                              # "> Nb >"
                              # "> State >"
                              # "> ExpandedKez(w)(2D) >"
                              n309 = case shown="\"Init\", Default" w821 {
                                tunnel: w820 -> [w834 _]
                                tunnel: w819 -> [w832 _]
                                tunnel: [w829 w882] -> w818
                                tunnel: w817 -> [_ w882]
                                tunnel: [w828 w875] -> w816
                                tunnel: w815 -> [_ w876]
                                tunnel: [w822 w883] -> w814
                                tunnel: w813 -> [_ w883]
                                tunnel: [w826 w881] -> w812
                                tunnel: w811 -> [_ w881]
                                tunnel: [_ w878] -> w810
                                tunnel: [enum16{"Init", "Mix rows"}."Mix rows" ("Cipher Phases") _] -> w809
                                tunnel: [FALSE TRUE] -> w808
                                tunnel: w807 -> [w822 _]
                                frame "Init", Default {
                                # "> Nb >"
                                # "> ExpandedKey(w)(2D) >"
                                # "> Nr >"
                                n310 = Reshape Array(w834, 60 ("dimension size"), 4 ("dimension size")) -> (w829:u32[][])
                                n311 = for {
                                N: 16 -> [_]
                                tunnel: w832 -> [w869]
                                shift-right: [w867] -> w830
                                shift-left: u16[][] [[0, 0, 0, 0], [0, 0, 0, 0], [0, 0, 0, 0], [0, 0, 0, 0]] ("State.Out") -> [w868]
                                i -> [w874]
                                n312 = Quotient & Remainder(x=w874, y=4) -> (x-y*floor(x/y)=w871:i32, floor(x/y)=w870:i32)
                                n313 = Index Array(array=w869, index=w874) -> (element=w872:u32)
                                n314 = Replace Array Subset(array=w868, new element=w872, index (row)=w871, index (col)=w870) -> (w867:u16[][])
                                }
                                n315 = Array Size(array=w829) -> (size(s)=w835:i32[])
                                n316 = Index Array(array=w835, index=0) -> (element=w838:i32)
                                n317 = Divide(x=w838, y=w822) -> (x/y=w837:dbl)
                                n318 = Decrement(x=w837) -> (x-1=w827:dbl)
                                n319 = To Long Integer(number=w827) -> (32bit integer=w826:i32)
                                n320 = stacked-sequence {
                                tunnel: w829 -> [w841]
                                tunnel: w822 -> [w843]
                                tunnel: w830 -> [w845]
                                tunnel: [w846] -> w828
                                tunnel: 0 ("rnd (0)") -> [w844]
                                frame #0 {
                                n321 = for {
                                N: 4 -> [_]
                                tunnel: w845 -> [w852]
                                tunnel: w841 -> [w851]
                                tunnel: w843 -> [w850]
                                tunnel: w844 -> [w849]
                                shift-right: [w847] -> w846
                                shift-left: w845 -> [w848]
                                i -> [w853]
                                # "w"
                                # "state"
                                # "r"
                                n322 = for {
                                N: w850 -> [_]
                                tunnel: w853 -> [w858]
                                tunnel: w852 -> [w861]
                                tunnel: w851 -> [w866]
                                tunnel: w849 -> [w865]
                                shift-right: [w854] -> w847
                                shift-left: w848 -> [w855]
                                i -> [w857]
                                # "c"
                                n323 = Multiply(x=w865, y=4) -> (x*y=w863:i32)
                                n324 = Add(x=w863, y=w857) -> (x+y=w862:i32)
                                n325 = Index Array(array=w861, index (row)=w858, index (col)=w857) -> (element=w860:u16)
                                n326 = Index Array(array=w866, index (row)=w862, index (col)=w858) -> (element=w859:u32)
                                n327 = Exclusive Or(1:w859, 2:w860) -> (0:w856:u32)
                                n328 = Replace Array Subset(array=w855, new element=w856, index (row)=w858, index (col)=w857) -> (w854:u16[][])
                                }
                                }
                                }
                                }
                                }
                                frame "Mix rows" {
                                # "var output : Array = new Array(4 * Nb); \n\tfor (var i : int = 0;i < 4 * Nb;i++)\n   {\n    output[i] = state[i % 4][Math.floor(i / 4)];\n\t\t\t}"
                                n329 = Decrement(x=w881) -> (x-1=w889:i32)
                                n330 = for {
                                N: w889 -> [_]
                                shift-right: [w972] -> w884
                                shift-left: w876 -> [w973]
                                tunnel: w883 -> [w971]
                                tunnel: w882 -> [w970]
                                i -> [w975]
                                # "round"
                                n331 = stacked-sequence {
                                tunnel: w971 -> [w979]
                                tunnel: w973 -> [w981]
                                tunnel: [w982] -> w978
                                frame #0 {
                                n332 = for {
                                N: 4 -> [_]
                                tunnel: w981 -> [w986]
                                shift-right: [w983] -> w982
                                shift-left: w981 -> [w985]
                                tunnel: w979 -> [w984]
                                i -> [w987]
                                # "> State.In >"
                                # "> State.Temp >"
                                # "r"
                                n333 = for {
                                N: w984 -> [_]
                                tunnel: w986 -> [w995]
                                tunnel: w987 -> [w992]
                                shift-right: [w988] -> w983
                                shift-left: w985 -> [w989]
                                i -> [w991]
                                # "Sbox"
                                # "s[r][c]"
                                # "c"
                                n334 = Index Array(array=w995, index (row)=w991, index (col)=w992) -> (element=w994:u16)
                                n335 = Index Array(array=u16[] [99, 124, 119, 123, 242, 107, 111, 197, 48, 1, 103, 43, 254, 215, 171, 118, 202, 130, 201, 125, 250, 89, 71, 240, 173, 212, 162, 175, 156, 164, 114, 192, 183, 253, 147, 38, 54, 63, 247, 204, 52, 165, 229, 241, 113, 216, 49, 21, 4, 199, 35, 195, 24, 150, 5, 154, 7, 18, 128, 226, 235, 39, 178, 117, 9, 131, 44, 26, 27, 110, 90, 160, 82, 59, 214, 179, 41, 227, 47, 132, 83, 209, 0, 237, 32, 252, 177, 91, 106, 203, 190, 57, 74, 76, 88, 207, 208, 239, 170, 251, 67, 77, 51, 133, 69, 249, 2, 127, 80, 60, 159, 168, 81, 163, 64, 143, 146, 157, 56, 245, 188, 182, 218, 33, 16, 255, 243, 210, 205, 12, 19, 236, 95, 151, 68, 23, 196, 167, 126, 61, 100, 93, 25, 115, 96, 129, 79, 220, 34, 42, 144, 136, 70, 238, 184, 20, 222, 94, 11, 219, 224, 50, 58, 10, 73, 6, 36, 92, 194, 211, 172, 98, 145, 149, 228, 121, 231, 200, 55, 109, 141, 213, 78, 169, 108, 86, 244, 234, 101, 122, 174, 8, 186, 120, 37, 46, 28, 166, 180, 198, 232, 221, 116, 31, 75, 189, 139, 138, 112, 62, 181, 102, 72, 3, 246, 14, 97, 53, 87, 185, 134, 193, 29, 158, 225, 248, 152, 17, 105, 217, 142, 148, 155, 30, 135, 233, 206, 85, 40, 223, 140, 161, 137, 13, 191, 230, 66, 104, 65, 153, 45, 15, 176, 84, 187, 22] ("Sbox"), index=w994) -> (element=w993:u16)
                                n336 = Replace Array Subset(array=w989, new element=w993, index (row)=w991, index (col)=w992) -> (w988:u16[][])
                                }
                                }
                                }
                                }
                                n337 = Increment(x=w975) -> (x+1=w974:i32)
                                n338 = stacked-sequence {
                                tunnel: w971 -> [w996]
                                tunnel: w978 -> [w998]
                                tunnel: [w999] -> w977
                                frame #0 {
                                n339 = for {
                                N: 3 -> [_]
                                tunnel: w998 -> [w1009]
                                shift-right: [w1005] -> w999
                                shift-left: w998 -> [w1006]
                                tunnel: w996 -> [w1000]
                                i -> [w1008]
                                # "> t[c] >"
                                # "> State.In >"
                                # "> State.Temp >"
                                # "r"
                                n340 = Increment(x=w1008) -> (x+1=w1007:i32)
                                n341 = for {
                                N: 4 -> [_]
                                tunnel: w1009 -> [w1024]
                                tunnel: w1007 -> [w1020]
                                shift-right: [w1016] -> w1003
                                shift-left: i32[] [0, 0, 0, 0] ("t[c]") -> [w1017]
                                tunnel: w1000 -> [w1022]
                                i -> [w1019]
                                # "c"
                                n342 = Add(x=w1020, y=w1019) -> (x+y=w1023:i32)
                                n343 = Quotient & Remainder(x=w1023, y=w1022) -> (x-y*floor(x/y)=w1021:i32)  [unwired: 1 out]
                                n344 = Index Array(array=w1024, index (row)=w1020, index (col)=w1021) -> (element=w1018:u16)
                                n345 = Insert Into Array(array=w1017, index=w1019, new element=w1018) -> (w1016:i32[])
                                }
                                n346 = for {
                                N: 4 -> [_]
                                tunnel: w1007 -> [w1015]
                                shift-right: [w1011] -> w1005
                                shift-left: w1006 -> [w1012]
                                tunnel: w1003 -> [w1010]
                                i -> [w1014]
                                # "c"
                                n347 = Index Array(array=w1010, index=w1014) -> (element=w1013:i32)
                                n348 = Replace Array Subset(array=w1012, new element=w1013, index (row)=w1015, index (col)=w1014) -> (w1011:u16[][])
                                }
                                }
                                }
                                }
                                n349 = stacked-sequence {
                                tunnel: w977 -> [w1026]
                                tunnel: [w1027] -> w976
                                frame #0 {
                                n350 = for {
                                N: 4 -> [_]
                                shift-right: [w1071] -> w1027
                                shift-left: w1026 -> [w1072]
                                tunnel: w1026 -> [w1073]
                                i -> [w1074]
                                # "> b >"
                                # "> a >"
                                # "> State.In >"
                                # "> State.Temp >"
                                # "c"
                                n351 = To Unsigned Word Integer(number=i32[] [0, 0, 0, 0] ("t[c]")) -> (unsigned 16bit integer=w1068:u16[])
                                n352 = To Unsigned Word Integer(number=i32[] [0, 0, 0, 0] ("t[c]")) -> (unsigned 16bit integer=w1067:u16[])
                                n353 = for {
                                N: 4 -> [_]
                                tunnel: w1073 -> [w1091]
                                tunnel: w1074 -> [w1090]
                                shift-right: [w1077] -> w1066
                                shift-left: w1068 -> [w1078]
                                shift-right: [w1075] -> w1065
                                shift-left: w1067 -> [w1076]
                                i -> [w1089]
                                # "s[i][c]"
                                # "i"
                                n354 = Index Array(array=w1091, index (row)=w1089, index (col)=w1090) -> (element=w1083:u16)
                                n355 = And(x=w1083, y=u16 128 ("0x80")) -> (x .and. y?=w1086:u16)
                                n356 = Logical Shift(y=i8 1, x=w1083) -> (x << y=w1080:u16)
                                n357 = Number To Boolean Array(number=w1086) -> (Boolean array=w1085:bool[])
                                n358 = Insert Into Array(array=w1078, index=w1089, new element=w1083) -> (w1077:u16[])
                                n359 = Exclusive Or(1:u16 283 ("0x011b"), 2:w1080) -> (0:w1081:u16)
                                n360 = Or Array Elements(Boolean array=w1085) -> (logical OR=w1084:bool)
                                n361 = Select(t=w1081, s=w1084, f=w1080) -> (s? t:f=w1088:u16)
                                n362 = Insert Into Array(array=w1076, index=w1089, new element=w1088) -> (w1075:u16[])
                                }
                                n363 = Index Array(array=w1065, index #1=0 ("index"), index #2=1 ("index"), index #3=2 ("index"), index #4=3 ("index")) -> (element #1=w1036:u16, element #2=w1048:u16, element #3=w1043:u16, element #4=w1033:u16)
                                n364 = Index Array(array=w1066, index #1=0 ("index"), index #2=1 ("index"), index #3=2 ("index"), index #4=3 ("index")) -> (element #1=w1037:u16, element #2=w1035:u16, element #3=w1034:u16, element #4=w1042:u16)
                                n365 = Exclusive Or(1:w1035, 2:w1036) -> (0:w1055:u16)
                                n366 = Exclusive Or(1:w1048, 2:w1055) -> (0:w1054:u16)
                                n367 = Exclusive Or(1:w1035, 2:w1037) -> (0:w1046:u16)
                                n368 = Exclusive Or(1:w1034, 2:w1054) -> (0:w1053:u16)
                                n369 = Exclusive Or(1:w1036, 2:w1037) -> (0:w1040:u16)
                                n370 = Exclusive Or(1:w1048, 2:w1037) -> (0:w1051:u16)
                                n371 = Exclusive Or(1:w1043, 2:w1046) -> (0:w1045:u16)
                                n372 = Exclusive Or(1:w1042, 2:w1053) -> (0:w1052:u16)
                                n373 = Exclusive Or(1:w1035, 2:w1040) -> (0:w1039:u16)
                                n374 = Exclusive Or(1:w1034, 2:w1051) -> (0:w1050:u16)
                                n375 = Exclusive Or(1:w1042, 2:w1045) -> (0:w1044:u16)
                                n376 = Exclusive Or(1:w1034, 2:w1039) -> (0:w1038:u16)
                                n377 = Exclusive Or(1:w1043, 2:w1050) -> (0:w1049:u16)
                                n378 = Exclusive Or(1:w1033, 2:w1044) -> (0:w1041:u16)
                                n379 = Exclusive Or(1:w1033, 2:w1038) -> (0:w1032:u16)
                                n380 = Exclusive Or(1:w1042, 2:w1049) -> (0:w1047:u16)
                                n381 = Replace Array Subset(array=w1072, new element #1=w1052, index (row) #1=0 ("disabled index (col)"), index (col) #1=w1074, new element #2=w1047, index (row) #2=1 ("disabled index (col)"), index (col) #2=w1074, new element #3=w1041, index (row) #3=2 ("disabled index (col)"), index (col) #3=w1074, new element #4=w1032, index (row) #4=3 ("disabled index (col)"), index (col) #4=w1074) -> (w1071:u16[][])
                                }
                                }
                                }
                                n382 = stacked-sequence {
                                tunnel: w970 -> [w1092]
                                tunnel: w971 -> [w1094]
                                tunnel: w976 -> [w1096]
                                tunnel: [w1097] -> w972
                                tunnel: w974 -> [w1095]
                                frame #0 {
                                n383 = for {
                                N: 4 -> [_]
                                tunnel: w1096 -> [w1103]
                                tunnel: w1092 -> [w1102]
                                tunnel: w1094 -> [w1101]
                                tunnel: w1095 -> [w1100]
                                shift-right: [w1098] -> w1097
                                shift-left: w1096 -> [w1099]
                                i -> [w1104]
                                # "w"
                                # "state"
                                # "r"
                                n384 = for {
                                N: w1101 -> [_]
                                tunnel: w1104 -> [w1109]
                                tunnel: w1103 -> [w1112]
                                tunnel: w1102 -> [w1117]
                                tunnel: w1100 -> [w1116]
                                shift-right: [w1105] -> w1098
                                shift-left: w1099 -> [w1106]
                                i -> [w1108]
                                # "c"
                                n385 = Multiply(x=w1116, y=4) -> (x*y=w1114:i32)
                                n386 = Add(x=w1114, y=w1108) -> (x+y=w1113:i32)
                                n387 = Index Array(array=w1112, index (row)=w1109, index (col)=w1108) -> (element=w1111:u16)
                                n388 = Index Array(array=w1117, index (row)=w1113, index (col)=w1109) -> (element=w1110:u32)
                                n389 = Exclusive Or(1:w1110, 2:w1111) -> (0:w1107:u32)
                                n390 = Replace Array Subset(array=w1106, new element=w1107, index (row)=w1109, index (col)=w1108) -> (w1105:u16[][])
                                }
                                }
                                }
                                }
                                }
                                n391 = stacked-sequence {
                                tunnel: w883 -> [w945]
                                tunnel: w884 -> [w947]
                                tunnel: [w948] -> w888
                                frame #0 {
                                n392 = for {
                                N: 4 -> [_]
                                tunnel: w947 -> [w952]
                                shift-right: [w949] -> w948
                                shift-left: w947 -> [w951]
                                tunnel: w945 -> [w950]
                                i -> [w953]
                                # "> State.In >"
                                # "> State.Temp >"
                                # "r"
                                n393 = for {
                                N: w950 -> [_]
                                tunnel: w952 -> [w961]
                                tunnel: w953 -> [w958]
                                shift-right: [w954] -> w949
                                shift-left: w951 -> [w955]
                                i -> [w957]
                                # "Sbox"
                                # "s[r][c]"
                                # "c"
                                n394 = Index Array(array=w961, index (row)=w957, index (col)=w958) -> (element=w960:u16)
                                n395 = Index Array(array=u16[] [99, 124, 119, 123, 242, 107, 111, 197, 48, 1, 103, 43, 254, 215, 171, 118, 202, 130, 201, 125, 250, 89, 71, 240, 173, 212, 162, 175, 156, 164, 114, 192, 183, 253, 147, 38, 54, 63, 247, 204, 52, 165, 229, 241, 113, 216, 49, 21, 4, 199, 35, 195, 24, 150, 5, 154, 7, 18, 128, 226, 235, 39, 178, 117, 9, 131, 44, 26, 27, 110, 90, 160, 82, 59, 214, 179, 41, 227, 47, 132, 83, 209, 0, 237, 32, 252, 177, 91, 106, 203, 190, 57, 74, 76, 88, 207, 208, 239, 170, 251, 67, 77, 51, 133, 69, 249, 2, 127, 80, 60, 159, 168, 81, 163, 64, 143, 146, 157, 56, 245, 188, 182, 218, 33, 16, 255, 243, 210, 205, 12, 19, 236, 95, 151, 68, 23, 196, 167, 126, 61, 100, 93, 25, 115, 96, 129, 79, 220, 34, 42, 144, 136, 70, 238, 184, 20, 222, 94, 11, 219, 224, 50, 58, 10, 73, 6, 36, 92, 194, 211, 172, 98, 145, 149, 228, 121, 231, 200, 55, 109, 141, 213, 78, 169, 108, 86, 244, 234, 101, 122, 174, 8, 186, 120, 37, 46, 28, 166, 180, 198, 232, 221, 116, 31, 75, 189, 139, 138, 112, 62, 181, 102, 72, 3, 246, 14, 97, 53, 87, 185, 134, 193, 29, 158, 225, 248, 152, 17, 105, 217, 142, 148, 155, 30, 135, 233, 206, 85, 40, 223, 140, 161, 137, 13, 191, 230, 66, 104, 65, 153, 45, 15, 176, 84, 187, 22] ("Sbox"), index=w960) -> (element=w959:u16)
                                n396 = Replace Array Subset(array=w955, new element=w959, index (row)=w957, index (col)=w958) -> (w954:u16[][])
                                }
                                }
                                }
                                }
                                n397 = stacked-sequence {
                                tunnel: w883 -> [w916]
                                tunnel: w888 -> [w918]
                                tunnel: [w919] -> w887
                                frame #0 {
                                n398 = for {
                                N: 3 -> [_]
                                tunnel: w918 -> [w929]
                                shift-right: [w925] -> w919
                                shift-left: w918 -> [w926]
                                tunnel: w916 -> [w920]
                                i -> [w928]
                                # "> t[c] >"
                                # "> State.In >"
                                # "> State.Temp >"
                                # "r"
                                n399 = Increment(x=w928) -> (x+1=w927:i32)
                                n400 = for {
                                N: 4 -> [_]
                                tunnel: w929 -> [w944]
                                tunnel: w927 -> [w940]
                                shift-right: [w936] -> w923
                                shift-left: i32[] [0, 0, 0, 0] ("t[c]") -> [w937]
                                tunnel: w920 -> [w942]
                                i -> [w939]
                                # "c"
                                n401 = Add(x=w940, y=w939) -> (x+y=w943:i32)
                                n402 = Quotient & Remainder(x=w943, y=w942) -> (x-y*floor(x/y)=w941:i32)  [unwired: 1 out]
                                n403 = Index Array(array=w944, index (row)=w940, index (col)=w941) -> (element=w938:u16)
                                n404 = Insert Into Array(array=w937, index=w939, new element=w938) -> (w936:i32[])
                                }
                                n405 = for {
                                N: 4 -> [_]
                                tunnel: w927 -> [w935]
                                shift-right: [w931] -> w925
                                shift-left: w926 -> [w932]
                                tunnel: w923 -> [w930]
                                i -> [w934]
                                # "c"
                                n406 = Index Array(array=w930, index=w934) -> (element=w933:i32)
                                n407 = Replace Array Subset(array=w932, new element=w933, index (row)=w935, index (col)=w934) -> (w931:u16[][])
                                }
                                }
                                }
                                }
                                n408 = stacked-sequence {
                                tunnel: w882 -> [w890]
                                tunnel: w883 -> [w892]
                                tunnel: w887 -> [w894]
                                tunnel: [w895] -> w875
                                tunnel: w881 -> [w893]
                                frame #0 {
                                n409 = for {
                                N: 4 -> [_]
                                tunnel: w894 -> [w901]
                                tunnel: w890 -> [w900]
                                tunnel: w892 -> [w899]
                                tunnel: w893 -> [w898]
                                shift-right: [w896] -> w895
                                shift-left: w894 -> [w897]
                                i -> [w902]
                                # "w"
                                # "state"
                                # "r"
                                n410 = for {
                                N: w899 -> [_]
                                tunnel: w902 -> [w907]
                                tunnel: w901 -> [w910]
                                tunnel: w900 -> [w915]
                                tunnel: w898 -> [w914]
                                shift-right: [w903] -> w896
                                shift-left: w897 -> [w904]
                                i -> [w906]
                                # "c"
                                n411 = Multiply(x=w914, y=4) -> (x*y=w912:i32)
                                n412 = Add(x=w912, y=w906) -> (x+y=w911:i32)
                                n413 = Index Array(array=w910, index (row)=w907, index (col)=w906) -> (element=w909:u16)
                                n414 = Index Array(array=w915, index (row)=w911, index (col)=w907) -> (element=w908:u32)
                                n415 = Exclusive Or(1:w908, 2:w909) -> (0:w905:u32)
                                n416 = Replace Array Subset(array=w904, new element=w905, index (row)=w907, index (col)=w906) -> (w903:u16[][])
                                }
                                }
                                }
                                }
                                n417 = Multiply(x=4, y=w883) -> (x*y=w880:i32)
                                n418 = Initialize Array(u16 0 ("x"), w880) -> (w879:u16[])
                                n419 = for {
                                N: w880 -> [_]
                                shift-right: [w962] -> w878
                                shift-left: w879 -> [w963]
                                tunnel: w875 -> [w964]
                                i -> [w966]
                                n420 = Quotient & Remainder(x=w966, y=4) -> (x-y*floor(x/y)=w968:i32, floor(x/y)=w967:i32)
                                n421 = Index Array(array=w964, index (row)=w968, index (col)=w967) -> (element=w965:u16)
                                n422 = Replace Array Subset(array=w963, new element=w965, index=w966) -> (w962:u16[])
                                }
                                }
                              }
                            }
                          }
                          frame Error {
                          }
                        }
                      }
                    }
                    "cipherCntr" <- w789
                  }
                  frame "Combine Bytes" {
                    n423 = Index Array(array=w1148, index=w1149) -> (element=w1151:string)
                    n424 = String Length(string=w1151) -> (length=w1152:i32)
                    n425 = Initialize Array(0, w1152) -> (w1147:i32[])
                    "plaintxtByte" <- w1147
                    n426 = for {
                      N: w1152 -> [_]
                      tunnel: w1149 -> [_]
                      tunnel: w1151 -> [w1159]
                      shift-right: [w1157] -> w1154
                      shift-left: w1147 -> [w1156]
                      tunnel: w1146 -> [w1155]
                      i -> [w1158]
                      # "> plaintxtByte >"
                      n427 = String To Byte Array(string=w1159) -> (unsigned byte array=w1162:u8[])
                      n428 = Index Array(array=w1162, index=w1158) -> (element=w1161:u8)
                      n429 = Index Array(array=w1155, index=w1158) -> (element=w1163:u16)
                      n430 = Exclusive Or(1:w1161, 2:w1163) -> (0:w1160:u16)
                      n431 = Replace Array Subset(array=w1156, new element=w1160, index=w1158) -> (w1157:i32[])
                    }
                    n432 = Byte Array To String(unsigned byte array=w1154) -> (string=w1150:string)
                    n433 = Concatenate Strings(w1143, w1150) -> (w1144:string)
                  }
                }
              }
            }
          }
        }
        n434 = UTF-8 to Text(8:w64, 11:w67) -> (0:w65:errorcluster, 3:w66:string)
        n435 = String To Byte Array(string=w67) -> (unsigned byte array=→"unsigned byte.utf8":u8[])
        n436 = String To Byte Array(string=w66) -> (unsigned byte array=→"unsigned byte.text":u8[])
      }
    }
    frame Error {
    }
  }
  "error out" <- w4
  "DecryptedText.Out" <- w1
